vi "Do_ADAM_channel.vi"(4 "Scan Period":dbl format="%.2f", 5 "Previous Scan Value":dbl format="%.2f", 6 "Present scan array":dbl[](array[numeric]) format="%.2f", 7 "Value to Output":dbl format="%.2f", 8 "Ch Description":T1 {"Duty" format="%.0b"; "D" format="%#_5g"; "C" format="%#_5g"; "B" format="%#_5g"; "A" format="%#_5g"}, 9 "Ch names":string[](array[string])) -> (0 "Scan comment":string, 1 "Output":dbl format="%.3f")   [LabVIEW 2014]
uses:
  ADAM Client/Sub VIs/ADAM Controls/Ch_description_ADAM.ctl
  ADAM Client/Sub VIs/ADAM Controls/Module_type_ADAM.ctl
  ADAM Client/Sub VIs/ADAM Controls/Function_ADAM.ctl
  ADAM Client/Sub VIs/ADAM Controls/Channel_State.ctl
  ADAM Client/Sub VIs/ADAM Controls/Calib_type_ADAM.ctl
  ADAM Client/Sub VIs/ADAM Controls/Address.ctl
  ADAM Client/Sub VIs/ADAM Controls/Remember_value_mode.ctl
  ADAM Serial/Instrument drivers/Arduino/ctls_and_globals/Arduino tx msg cluster.ctl
  ADAM Client/Sub VIs/ADAM Controls/Search_mode.ctl
  Anemometry/Anemometry Sub Vis/Controls/In_Range.ctl
  <vilib>/Analysis/baseanly.llb/Mean (DBL).vi
  ADAM_Global.vi
  Anemometry/Anemometry Sub Vis/Globals/Gas_management_global.vi
  Anemometry/Anemometry Sub Vis/Globals/Constants_global.vi
  <vilib>/Analysis/NI_AALBase.lvlib
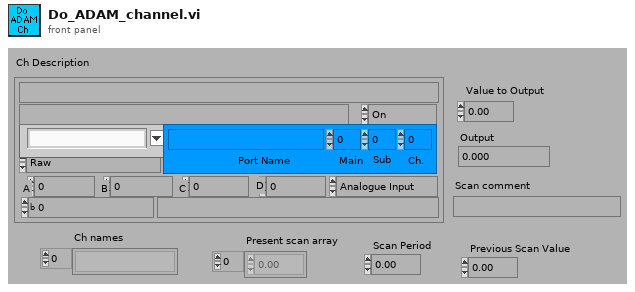
[diagram p1: front panel]
types:
  T1 = typedef "Ch_description_ADAM.ctl" = cluster{"Ch Name":string, "Type":T2, "Function":T3, "Ch State":T4, "Calibration type":T5, "A":dbl, "B":dbl, "C":dbl, "D":dbl, "Comments":string, "Address":T6, "String":string, "Duty":u16}
  T2 = typedef "Module_type_ADAM.ctl" = string
  T3 = typedef "Function_ADAM.ctl" = enum16{"Analogue Input", "Digital Input", "Event counter", "Event rate", "Analogue Output", "Digital Output", "Relay Output"}
  T4 = typedef "Channel_State.ctl" = enum16{"On", "Off", "Always On", "Always Off"}
  T5 = typedef "Calib_type_ADAM.ctl" = enum16{"Raw", "Bx + A", "Cx^2 + Bx + A", "Dx^3 + Cx^2 + Bx + A", "In Band", "Hi-Tec Q", "Hi-Tec M_dot", "Text"}
  T6 = typedef "Address.ctl" = cluster{"Main":i32, "Ch.":i32, "Sub":i32, "Port Name":string}
  T7 = typedef "Remember_value_mode.ctl" = enum16{"Read only", "Read and Write"}
  T8 = typedef "Search_mode.ctl" = enum16{"Between times", "All Times"}
  T9 = typedef "In_Range.ctl" = enum16{"%", "±", "% & ±"}
  T10 = typedef "Arduino tx msg cluster.ctl" = cluster{"dest":u8, "A/D/C/I":string, "R/W":string, "chan":u8, "val (float)":sgl}
  T11 = typedef "Client_State_Cluster.ctl" = cluster{"Client Name":string, "Traverse level State":T12, "People to Email":string[], "Next Contact Time":dbl}
  T12 = typedef "Traverse_Level_State.ctl" = enum16{"Running", "Complete"}
  T13 = cluster{"Centre Times":dbl[], "Output array":dbl[]}
  T14 = cluster{"Centre Times":dbl[], "Output array":dbl[]}[]
  T15 = typedef "Valco_valve_ph.ctl" = u16
  T16 = typedef "LVDateTimeRec.ctl" = cluster{"fractional second":dbl, "second":i32, "minute":i32, "hour":i32, "day of month":i32, "month":i32, "year":i32, "day of week":i32, "day of year":i32, "DST":i32}
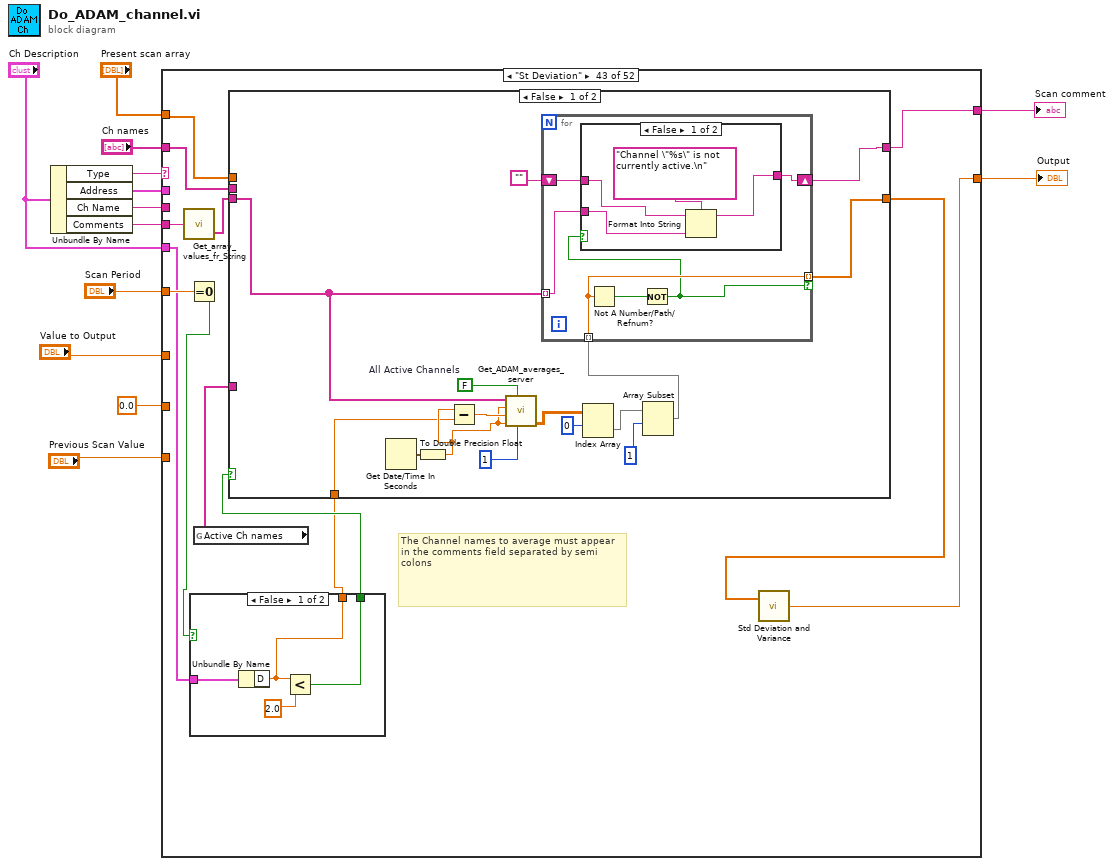
[diagram p0: block diagram]
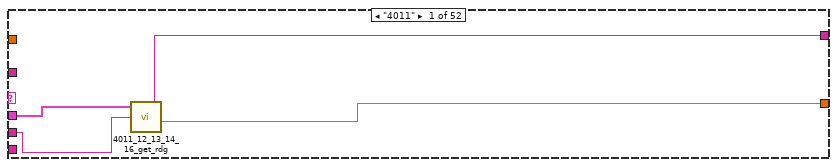
[diagram p2: hidden frame]
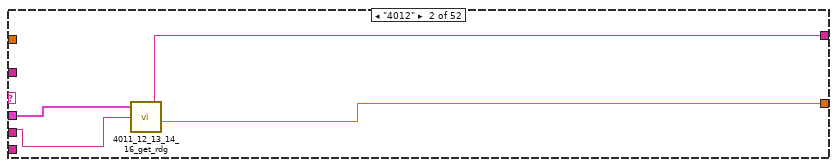
[diagram p3: hidden frame]
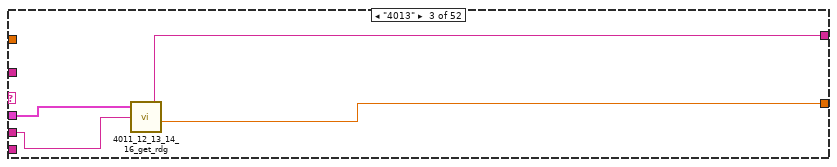
[diagram p4: hidden frame]
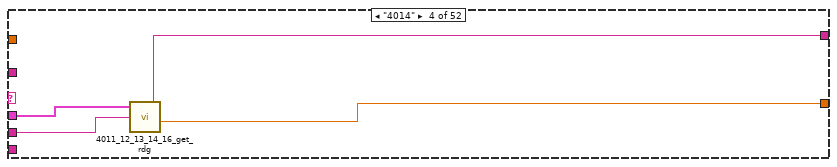
[diagram p5: hidden frame]
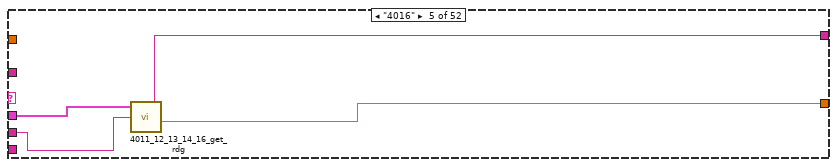
[diagram p6: hidden frame]
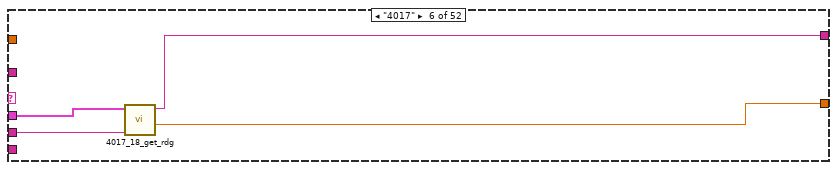
[diagram p7: hidden frame]
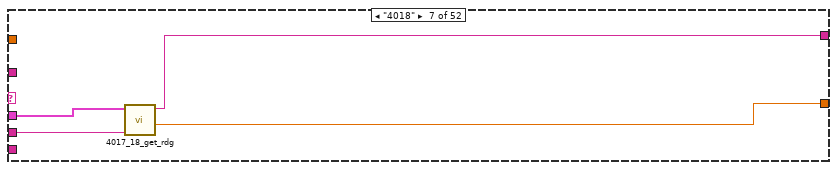
[diagram p8: hidden frame]
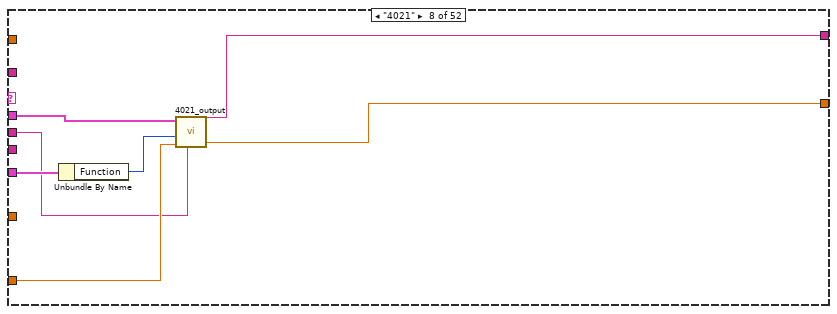
[diagram p9: hidden frame]
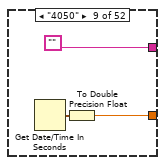
[diagram p10: hidden frame]
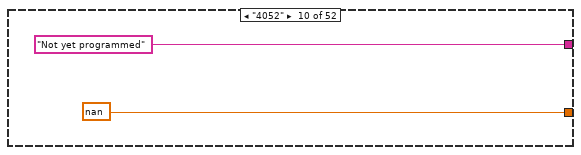
[diagram p11: hidden frame]
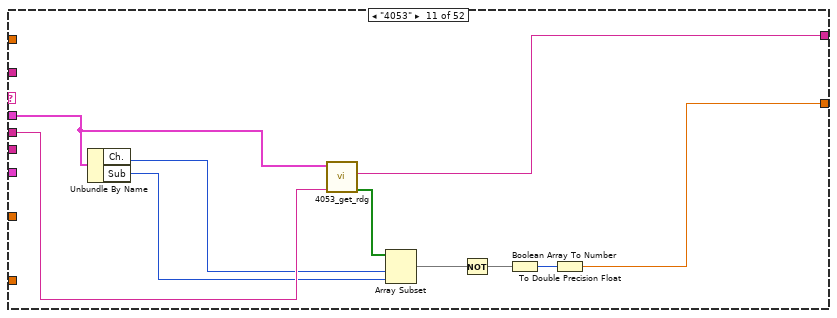
[diagram p12: hidden frame]
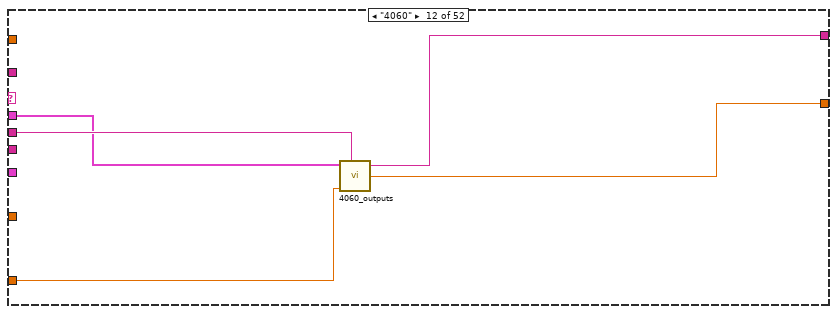
[diagram p13: hidden frame]
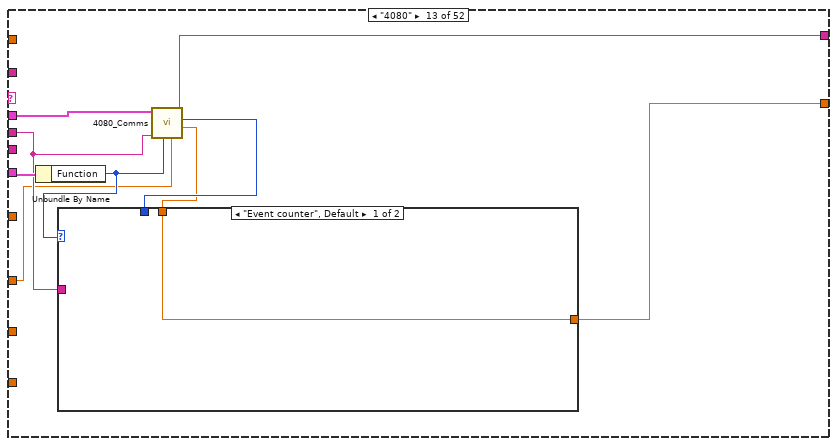
[diagram p14: hidden frame]
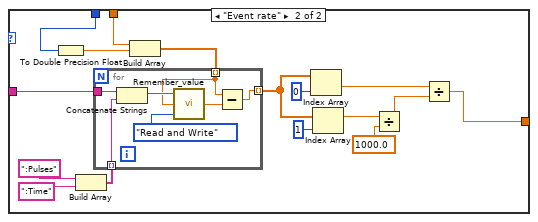
[diagram p15: hidden frame]
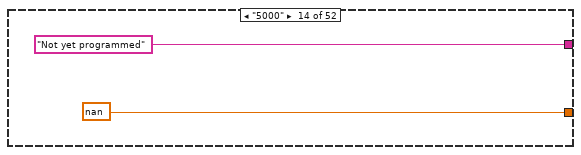
[diagram p16: hidden frame]
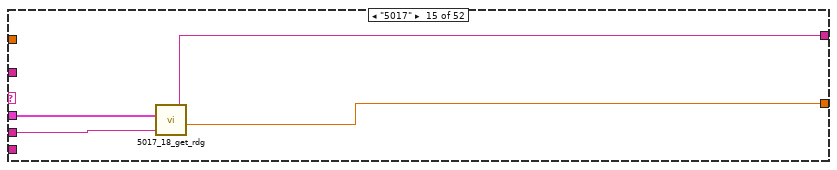
[diagram p17: hidden frame]
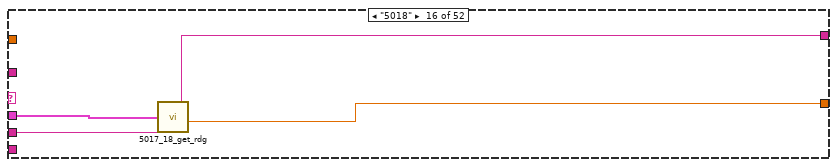
[diagram p18: hidden frame]
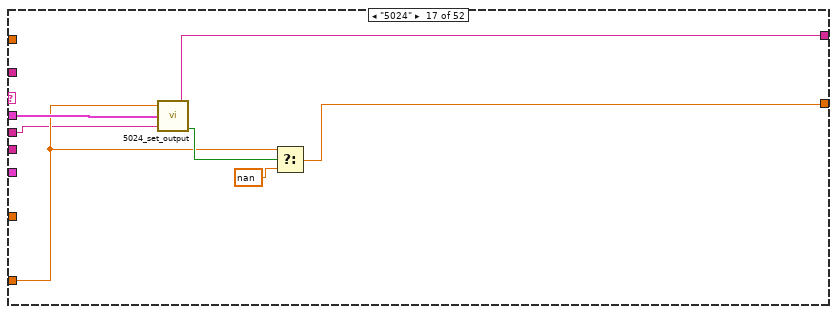
[diagram p19: hidden frame]
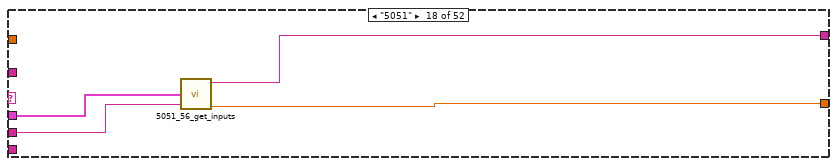
[diagram p20: hidden frame]
diagram:
  n1 = Unbundle By Name("Ch Description") -> ("Type"=w11:T2, "Address"=w10:T6, "Ch Name"=w2:string, "Comments"=w7:string)
  n2 = case shown="\"St Deviation\"" w11 {
    tunnel: [w16 w20 w24 w28 w32 w36 w40 w47 w50 nan w57 w66 w75 nan w105 w109 w114 w120 w128 w149 w171 w190 w205 w221 w250 w270 w358 w371 w373 w375 nan w483 w484 w487 w503 w515 0.0 ("Output") w524 w525 w529 w537 w568 w576 w659 w660 w666 w740 w788 w1279 nan w1310 w1336] -> w8
    tunnel: [w17 w21 w25 w29 w33 w37 w41 w48 "" "Not yet programmed" w62 w67 w77 "Not yet programmed" w106 w110 w117 w121 w127 w150 w172 w189 w208 w223 w245 w267 "" w372 "" w396 "Not yet programmed" w482 "" w488 w502 w516 "Warning; unmatched case in Do_ADAM_channel" ("Status note") w523 "" w530 w536 w567 w570 "Crazy time based random number!" w664 w668 w732 w787 w1280 "Not yet programmed" w1299 ""] -> w5
    tunnel: w10 -> [w14 w18 w22 w26 w30 w34 w38 w42 _ _ w54 w65 w69 _ w107 w111 w118 w122 w126 w151 w173 w204 w220 w236 w261 _ _ w370 _ _ _ w480 _ w486 w505 w518 _ w521 _ _ _ _ _ _ w662 w670 w737 w779 w1285 _ _ w1345]
    tunnel: "Ch Description" -> [_ _ _ _ _ _ _ w46 _ _ _ _ w76 _ _ _ _ _ w125 w148 w170 _ _ _ _ w274 _ _ _ w401 _ _ _ _ _ _ _ _ w526 w531 w542 w569 w574 _ _ w669 _ w781 _ _ _ _]
    tunnel: w2 -> [w15 w19 w23 w27 w31 w35 w39 w43 _ _ w63 w68 w72 _ w104 w108 w112 w119 w123 w145 w167 _ _ _ _ _ w354 _ _ _ _ w481 _ _ w504 w517 _ w522 _ _ _ _ _ _ w663 w667 w733 w784 w1284 _ w1306 _]
    tunnel: "Ch names" -> [_ _ _ _ _ _ _ _ _ _ _ _ _ _ _ _ _ _ _ _ _ _ _ _ _ w279 _ _ _ w400 _ _ _ _ _ _ _ _ _ w532 w543 _ w582 _ _ _ _ w786 _ _ _ _]
    tunnel: "Present scan array" -> [_ _ _ _ _ _ _ _ _ _ _ _ _ _ _ _ _ _ _ _ _ _ _ _ _ w278 _ _ _ w398 _ _ _ _ _ _ _ _ _ w533 w540 _ w581 _ _ _ _ w785 _ _ _ _]
    tunnel: w7 -> [_ _ _ _ _ _ _ _ _ _ _ _ _ _ _ _ _ _ _ _ _ _ _ _ _ w277 _ _ _ w402 _ _ _ _ _ _ _ _ _ _ w535 _ w580 _ _ _ _ _ _ _ _ _]
    tunnel: "Value to Output" -> [_ _ _ _ _ _ _ w44 _ _ _ w64 w70 _ _ _ w113 _ w124 w146 w168 _ w206 w222 _ _ _ _ _ _ _ _ _ _ w501 _ _ _ _ _ w541 _ _ _ _ w665 w741 _ _ _ _ w1340]
    tunnel: "Scan Period" -> [_ _ _ _ _ _ _ _ _ _ _ _ _ _ _ _ _ _ _ _ _ _ _ _ _ w269 _ _ _ _ _ _ _ _ _ _ _ _ _ _ w538 _ w575 _ _ _ _ w783 _ _ _ _]
    tunnel: "Previous Scan Value" -> [_ _ _ _ _ _ _ _ _ _ _ _ _ _ _ _ _ _ _ _ _ w192 _ _ w237 _ _ _ w373 w376 _ _ w484 _ _ _ _ _ _ _ w539 _ _ _ _ _ _ w782 _ _ _ _]
    tunnel: 0.0 -> [_ _ _ _ _ _ _ _ _ _ _ _ _ _ _ _ _ _ _ _ _ _ _ _ _ _ _ _ _ _ _ _ _ _ _ _ _ _ _ _ _ _ _ _ _ _ _ w780 _ _ _ _]
    frame "4011" {
      n3 = call "4011_12_13_14_16_get_rdg.vi"("Address"=w14, "Channel Name"=w15) -> ("Comment"=w17:string, "Reading"=w16:dbl)  [unwired: 1 in, 2 out]
    }
    frame "4012" {
      n4 = call "4011_12_13_14_16_get_rdg.vi"("Address"=w18, "Channel Name"=w19) -> ("Comment"=w21:string, "Reading"=w20:dbl)  [unwired: 1 in, 2 out]
    }
    frame "4013" {
      n5 = call "4011_12_13_14_16_get_rdg.vi"("Address"=w22, "Channel Name"=w23) -> ("Comment"=w25:string, "Reading"=w24:dbl)  [unwired: 1 in, 2 out]
    }
    frame "4014" {
      n6 = call "4011_12_13_14_16_get_rdg.vi"("Address"=w26, "Channel Name"=w27) -> ("Comment"=w29:string, "Reading"=w28:dbl)  [unwired: 1 in, 2 out]
    }
    frame "4016" {
      n7 = call "4011_12_13_14_16_get_rdg.vi"("Address"=w30, "Channel Name"=w31) -> ("Comment"=w33:string, "Reading"=w32:dbl)  [unwired: 1 in, 2 out]
    }
    frame "4017" {
      n8 = call "4017_18_get_rdg.vi"("Channel Name"=w35, "Address"=w34) -> ("Reading"=w36:dbl, "Comment"=w37:string)  [unwired: 2 in, 2 out]
    }
    frame "4018" {
      n9 = call "4017_18_get_rdg.vi"("Channel Name"=w39, "Address"=w38) -> ("Reading"=w40:dbl, "Comment"=w41:string)  [unwired: 2 in, 2 out]
    }
    frame "4021" {
      n10 = Unbundle By Name(w46) -> ("Function"=w45:T3)
      n11 = call "4021_output.vi"("Address"=w42, "Function"=w45, "Set to:"=w44, "Channel Name"=w43) -> ("Comment"=w48:string, "Reading"=w47:dbl)  [unwired: 1 in, 1 out]
    }
    frame "4050" {
      n12 = Get Date/Time In Seconds() -> (seconds since 1Jan1904=w49:timestamp)
      n13 = To Double Precision Float(number=w49) -> (double precision float=w50:dbl)
    }
    frame "4052" {
    }
    frame "4053" {
      n14 = Unbundle By Name(w54) -> ("Ch."=w55:i32, "Sub"=w61:i32)
      n15 = call "4053_get_rdg.vi"("Channel Name"=w63, "Address"=w54) -> ("Boolean array"=w60:bool[], "Comment"=w62:string)  [unwired: 2 in, 2 out]
      n16 = Array Subset(array=w60, index=w55, length=w61) -> (w59:bool[])
      n17 = Not(x=w59) -> (.not. x?=w56:bool[])
      n18 = Boolean Array To Number(Boolean array=w56) -> (number=w58:u32)
      n19 = To Double Precision Float(number=w58) -> (double precision float=w57:dbl)
    }
    frame "4060" {
      n20 = call "4060_outputs.vi"("Address"=w65, "Value to Output"=w64, "Channel Name"=w68) -> ("Comment"=w67:string, "Reading"=w66:dbl)  [unwired: 2 in, 1 out]
    }
    frame "4080" {
      n21 = Unbundle By Name(w76) -> ("Function"=w71:T3)
      n22 = call "4080_Comms.vi"("Value to display"=w70, "Function"=w71, "Channel Name"=w72, "Address"=w69) -> ("Reading"=w73:dbl, "millisecond timer value"=w74:u32, "Comment"=w77:string)  [unwired: 2 in, 1 out]
      n23 = case shown="\"Event counter\", Default" w71 {
        tunnel: w72 -> [_ w94]
        tunnel: w74 -> [_ w87]
        tunnel: [w78 w79] -> w75
        tunnel: w73 -> [w78 w88]
        frame "Event counter", Default {
        }
        frame "Event rate" {
          n24 = To Double Precision Float(number=w87) -> (double precision float=w86:dbl)
          n25 = Build Array(":Pulses", ":Time") -> (w89:string[])
          n26 = Build Array(w88, w86) -> (w85:dbl[])
          n27 = for {
            tunnel: w94 -> [w98]
            tunnel: [w99] -> w82 mode=indexing
            tunnel: w89 -> [w96] mode=indexing
            tunnel: w85 -> [w95] mode=indexing
            n28 = Concatenate Strings(w98, w96) -> (w97:string)
            n29 = call "Remember_value.vi"("Mode"=Remember_value_mode."Read and Write", "Input Value"=w95, "Ch name"=w97) -> ("Output Value"=w100:dbl)
            n30 = Subtract(x=w95, y=w100) -> (x-y=w99:dbl)
          }
          n31 = Index Array(array=w82, index=0) -> (element=w80:dbl)
          n32 = Index Array(array=w82, index=1) -> (element=w81:dbl)
          n33 = Divide(x=w81, y=1000.0) -> (x/y=w92:dbl)
          n34 = Divide(x=w80, y=w92) -> (x/y=w79:dbl)
        }
      }
    }
    frame "5000" {
    }
    frame "5017" {
      n35 = call "5017_18_get_rdg.vi"("Address (all reqd.)"=w107, "Channel Name"=w104) -> ("Comment"=w106:string, "Reading"=w105:dbl)  [unwired: 3 out]
    }
    frame "5018" {
      n36 = call "5017_18_get_rdg.vi"("Address (all reqd.)"=w111, "Channel Name"=w108) -> ("Comment"=w110:string, "Reading"=w109:dbl)  [unwired: 3 out]
    }
    frame "5024" {
      n37 = call "5024_set_output.vi"("Set to:"=w113, "Address (all reqd.)"=w118, "Channel Name"=w112) -> ("Comment"=w117:string, "Good Reply"=w115:bool)  [unwired: 2 out]
      n38 = Select(t=w113, s=w115, f=nan) -> (s? t:f=w114:dbl)
    }
    frame "5051" {
      n39 = call "5051_56_get_inputs.vi"("Address (Main, Sub reqd.)"=w122, "Channel Name"=w119) -> ("Comment"=w121:string, "Single output"=w120:dbl)  [unwired: 3 out]
    }
    frame "5056" {
      n40 = Unbundle By Name(w125) -> ("Function"=w129:T3)
      n41 = case shown="\"Digital Input\"" w129 {
        tunnel: w126 -> [_ w135 w144]
        tunnel: ["This function is not available" w136 w142] -> w127
        tunnel: [nan ("A") w133 w139] -> w128
        tunnel: w124 -> [_ _ w138]
        tunnel: w123 -> [_ w132 w137]
        frame "Analogue Input", Default {
        }
        frame "Digital Input" {
          # "Readback value"
          n42 = call "5060_check_outputs.vi"("Address (Main, Sub reqd.)"=w135, "Channel Name"=w132) -> ("Comment"=w136:string, "Single Channel"=w134:i16)  [unwired: 3 out]
          n43 = To Double Precision Float(number=w134) -> (double precision float=w133:dbl)
        }
        frame "Relay Output" {
          # "Sets single o/p channel"
          n44 = Greater Than 0?(x=w138) -> (x > 0?=w143:bool)
          n45 = call "5056_60_set_single_output.vi"("Channel Name"=w137, "Address (all reqd.)"=w144, "Set state:"=w143) -> ("Comment"=w142:string, "Good Reply"=w141:bool)  [unwired: 2 out]
          n46 = Select(t=w138, s=w141, f=nan) -> (s? t:f=w139:dbl)
        }
      }
    }
    frame "5060" {
      n47 = Unbundle By Name(w148) -> ("Function"=w147:T3)
      n48 = case shown="\"Relay Output\"" w147 {
        tunnel: w151 -> [_ w157 w166]
        tunnel: ["This function is not available" w158 w164] -> w150
        tunnel: [nan ("A") w155 w161] -> w149
        tunnel: w146 -> [_ _ w160]
        tunnel: w145 -> [_ w154 w159]
        frame "Analogue Input", Default {
        }
        frame "Digital Input" {
          # "Readback value"
          n49 = call "5060_check_outputs.vi"("Address (Main, Sub reqd.)"=w157, "Channel Name"=w154) -> ("Comment"=w158:string, "Single Channel"=w156:i16)  [unwired: 3 out]
          n50 = To Double Precision Float(number=w156) -> (double precision float=w155:dbl)
        }
        frame "Relay Output" {
          # "Sets single o/p channel"
          n51 = Greater Than 0?(x=w160) -> (x > 0?=w165:bool)
          n52 = call "5056_60_set_single_output.vi"("Channel Name"=w159, "Address (all reqd.)"=w166, "Set state:"=w165) -> ("Comment"=w164:string, "Good Reply"=w163:bool)  [unwired: 2 out]
          n53 = Select(t=w160, s=w163, f=nan) -> (s? t:f=w161:dbl)
        }
      }
    }
    frame "6060" {
      n54 = Unbundle By Name(w170) -> ("Function"=w169:T3)
      n55 = case shown="\"Digital Input\"" w169 {
        tunnel: w173 -> [_ w179 w188]
        tunnel: ["This function is not available" w180 w186] -> w172
        tunnel: [nan ("A") w177 w183] -> w171
        tunnel: w168 -> [_ _ w182]
        tunnel: w167 -> [_ w176 w181]
        frame "Analogue Input", Default {
        }
        frame "Digital Input" {
          n56 = call "6060_read_all_I-O.vi"("Address (Main, Sub reqd.)"=w179, "Channel Name"=w176) -> ("Comment"=w180:string, "Single Input Channel"=w178:i16)  [unwired: 3 out]
          n57 = To Double Precision Float(number=w178) -> (double precision float=w177:dbl)
        }
        frame "Relay Output" {
          # "Sets single o/p channel"
          n58 = Greater Than 0?(x=w182) -> (x > 0?=w187:bool)
          n59 = call "6060_set_single_output.vi"("Channel Name"=w181, "Address (Main, Ch requd.)"=w188, "Set state:"=w187) -> ("Comment"=w186:string, "Good Reply"=w185:bool)  [unwired: 2 out]
          n60 = Select(t=w182, s=w185, f=nan) -> (s? t:f=w183:dbl)
        }
      }
    }
    frame "Arduino A_in" {
      w198 = T10 {"dest"=1, "A/D/C/I"="A", "R/W"="R", "chan"=1, "val (float)"=0.0}  # Tx msg cluster
      # "Analogue read case"
      n61 = Unbundle By Name(w204) -> ("Port Name"=w195:string, "Main"=w196:i32, "Ch."=w197:i32)
      n62 = To Unsigned Byte Integer(number=w196) -> (unsigned 8bit integer=w203:u8)
      n63 = To Unsigned Byte Integer(number=w197) -> (unsigned 8bit integer=w201:u8)
      n64 = Bundle By Name(cluster=w198, "dest"=w203, "A/D/C/I"="A" ("A/D"), "R/W"="R", "chan"=w201, "val (float)"=sgl 0.0) -> (w194:T10)
      n65 = call "Arduino generic wrapper.vi"("Tx msg cluster"=w194, "Port name"=w195) -> ("Scan comment"=w189:string, "Output"=w191:dbl)
      n66 = Empty String/Path?(string/path=w189) -> (empty?=w193:bool)
      n67 = Select(t=w191, s=w193, f=w192) -> (s? t:f=w190:dbl)
    }
    frame "Arduino A_out" {
      w215 = T10 {"dest"=1, "A/D/C/I"="A", "R/W"="R", "chan"=1, "val (float)"=0.0}  # Tx msg cluster
      # "Analogue write case"
      n68 = Unbundle By Name(w220) -> ("Port Name"=w212:string, "Main"=w213:i32, "Ch."=w214:i32)
      n69 = To Unsigned Byte Integer(number=w213) -> (unsigned 8bit integer=w219:u8)
      n70 = To Unsigned Byte Integer(number=w214) -> (unsigned 8bit integer=w218:u8)
      n71 = To Single Precision Float(number=w206) -> (single precision float=w210:sgl)
      n72 = Bundle By Name(cluster=w215, "dest"=w219, "A/D/C/I"="A" ("A/D"), "R/W"="W", "chan"=w218, "val (float)"=w210) -> (w211:T10)
      n73 = call "Arduino generic wrapper.vi"("Tx msg cluster"=w211, "Port name"=w212) -> ("Scan comment"=w208:string)  [unwired: 1 out]
      n74 = Empty String/Path?(string/path=w208) -> (empty?=w207:bool)
      n75 = Select(t=w206, s=w207, f=nan ("Reading")) -> (s? t:f=w205:dbl)
    }
    frame "Arduino D_out" {
      w231 = T10 {"dest"=1, "A/D/C/I"="A", "R/W"="R", "chan"=1, "val (float)"=0.0}  # Tx msg cluster
      # "Digital write case"
      n76 = Unbundle By Name(w236) -> ("Port Name"=w228:string, "Main"=w229:i32, "Ch."=w230:i32)
      n77 = To Unsigned Byte Integer(number=w229) -> (unsigned 8bit integer=w235:u8)
      n78 = To Unsigned Byte Integer(number=w230) -> (unsigned 8bit integer=w234:u8)
      n79 = To Single Precision Float(number=w222) -> (single precision float=w226:sgl)
      n80 = Bundle By Name(cluster=w231, "dest"=w235, "A/D/C/I"="D" ("A/D"), "R/W"="W", "chan"=w234, "val (float)"=w226) -> (w227:T10)
      n81 = call "Arduino generic wrapper.vi"("Tx msg cluster"=w227, "Port name"=w228) -> ("Scan comment"=w223:string)  [unwired: 1 out]
      n82 = Empty String/Path?(string/path=w223) -> (empty?=w224:bool)
      n83 = Select(t=w222, s=w224, f=nan ("Reading")) -> (s? t:f=w221:dbl)
    }
    frame "Arduino Thermistor" {
      w255 = T10 {"dest"=1, "A/D/C/I"="A", "R/W"="R", "chan"=1, "val (float)"=0.0}  # Tx msg cluster
      # "Thermistor read case"
      # "values not expected in 'normal' operating conditions"
      n84 = Unbundle By Name(w261) -> ("Port Name"=w252:string, "Main"=w253:i32, "Ch."=w254:i32)
      n85 = To Unsigned Byte Integer(number=w253) -> (unsigned 8bit integer=w260:u8)
      n86 = To Unsigned Byte Integer(number=w254) -> (unsigned 8bit integer=w258:u8)
      n87 = Bundle By Name(cluster=w255, "dest"=w260, "A/D/C/I"="A" ("A/D"), "R/W"="R", "chan"=w258, "val (float)"=sgl 0.0) -> (w251:T10)
      n88 = call "Arduino generic wrapper.vi"("Tx msg cluster"=w251, "Port name"=w252) -> ("Scan comment"=w241:string, "Output"=w239:dbl)
      n89 = Empty String/Path?(string/path=w241) -> (empty?=w240:bool)
      n90 = Select(t=w239, s=w240, f=w237) -> (s? t:f=w238:dbl)
      n91 = Less?(x=w239, y=-40.0) -> (x < y?=w242:bool)
      n92 = Greater?(x=w239, y=140.0) -> (0:w243:bool)
      n93 = case shown="False" w242 {
        tunnel: [w263 "Faulty thermistor open-circuit;"] -> w244
        tunnel: w243 -> [w262 _]
        frame False {
          n94 = case shown="True" w262 {
            tunnel: ["" "Faulty thermistor short-circuit;"] -> w263
            frame False {
            }
            frame True {
            }
          }
        }
        frame True {
        }
      }
      n95 = Or(x=w242, y=w243) -> (x .or. y?=w247:bool)
      n96 = Select(t=nan ("f"), s=w247, f=w238) -> (s? t:f=w250:dbl)
      n97 = Concatenate Strings(w241, w244) -> (w245:string)
    }
    frame "Average" {
      # "The Channel names to average must appear in the comments field separated by semi colons"
      n98 = call "Get_array_values_fr_String.vi"("String Value"=w277) -> ("String array"=w276:string[])  [unwired: 1 out]
      n99 = Equal To 0?(x=w269) -> (x = 0?=w268:bool)
      n100 = global read "ADAM_Global.vi" "Active Ch names"() -> (w275:string[])
      n101 = case shown="False" w268 {
        tunnel: w274 -> [w283 _]
        tunnel: [w281 TRUE] -> w273
        tunnel: [w280 2.0 ("A")] -> w272
        frame False {
          n102 = Unbundle By Name(w283) -> ("D"=w280:dbl)
          n103 = Less?(x=w280, y=2.0) -> (x < y?=w281:bool)
        }
        frame True {
        }
      }
      n104 = case shown="True" w273 {
        tunnel: w279 -> [_ w318]
        tunnel: w278 -> [_ w317]
        tunnel: w276 -> [w288 w316]
        tunnel: [w286 w314] -> w267
        tunnel: w275 -> [_ w313]
        tunnel: [w289 w312] -> w271
        tunnel: w272 -> [w290 _]
        frame False {
          w297 = FALSE  # All Active Channels
          n105 = Get Date/Time In Seconds() -> (seconds since 1Jan1904=w300:timestamp)
          n106 = To Double Precision Float(number=w300) -> (double precision float=w298:dbl)
          n107 = Subtract(x=w298, y=w290) -> (x-y=w299:dbl)
          n108 = call "Get_ADAM_averages_server.vi"("No of averages"=1, "All Active Channels"=w297, "End time"=w298, "Start time"=w299, "Clients time"=w298, "ADAM Ch Names"=w288) -> ("DBL values"=w295:dbl[][])  [unwired: 4 out]
          n109 = Index Array(array=w295, index (row)=0) -> (element=w292:dbl[])  [unwired: 1 in]
          n110 = Array Subset(array=w292, index=1) -> (w291:dbl[])  [unwired: 1 in]
          n111 = for {
            tunnel: w291 -> [w306] mode=indexing
            tunnel: [w306] -> w289 mode=indexing if=w304
            tunnel: w288 -> [w303] mode=indexing
            shift-right: [w301] -> w286
            shift-left: "" -> [w302]
            n112 = Not A Number/Path/Refnum?(number/path/refnum=w306) -> (NaN/Path/Refnum?=w305:bool)
            n113 = Not(x=w305) -> (.not. x?=w304:bool)
            n114 = case shown="False" w304 {
              tunnel: w303 -> [w309 _]
              tunnel: w302 -> [w308 w311]
              tunnel: [w307 w311] -> w301
              frame False {
                n115 = Format Into String(format string="Channel \"%s\" is not currently active.\n", initial string=w308, w309) -> (resulting string=w307:string)  [unwired: 1 in, 1 out]
              }
              frame True {
              }
            }
          }
        }
        frame True {
          n116 = for {
            tunnel: w318 -> [w331]
            tunnel: w317 -> [w330]
            tunnel: w316 -> [w327] mode=indexing
            shift-right: [w328] -> w314
            shift-left: "" -> [w329]
            tunnel: [w321] -> w312 mode=indexing if=w319
            tunnel: w313 -> [w322]
            n117 = call "Read_value_of_earlier_Ch.vi"("Desired Ch to Read"=w327, "Ch names"=w331, "Present scan array"=w330) -> ("Value"=w325:dbl, "Scan comment"=w324:string)  [unwired: 1 in]
            n118 = Not A Number/Path/Refnum?(number/path/refnum=w325) -> (NaN/Path/Refnum?=w326:bool)
            n119 = case shown="False" w326 {
              tunnel: w327 -> [w334 _]
              tunnel: [w337 w347] -> w321
              tunnel: w325 -> [w336 w347]
              tunnel: [w339 w346] -> w323
              tunnel: w324 -> [w338 w346]
              tunnel: w322 -> [w335 _]
              frame False {
                n120 = Search 1D Array(1D array=w335, element=w334) -> (index of element=w332:i32)  [unwired: 1 in]
                n121 = Greater Or Equal To 0?(x=w332) -> (x >= 0?=w333:bool)
                n122 = case shown="False" w333 {
                  tunnel: w334 -> [w343 _]
                  tunnel: [w342 w345] -> w339
                  tunnel: w338 -> [_ w345]
                  tunnel: [nan w344] -> w337
                  tunnel: w336 -> [_ w344]
                  frame False {
                    n123 = Format Into String(format string="Channel \"%s\" is not currently active.\n", w343) -> (resulting string=w342:string)  [unwired: 2 in, 1 out]
                  }
                  frame True {
                  }
                }
              }
              frame True {
              }
            }
            n124 = Concatenate Strings(w329, w323) -> (w328:string)
            n125 = Not A Number/Path/Refnum?(number/path/refnum=w321) -> (NaN/Path/Refnum?=w320:bool)
            n126 = Not(x=w320) -> (.not. x?=w319:bool)
          }
        }
      }
      n127 = call-poly <vilib>:"Mean.vi"("X"=w271) -> ("mean"=w270:dbl)  [unwired: 1 out]
    }
    frame "Client Info" {
      n128 = global read "ADAM_Global.vi" "Client State Array"() -> (w360:T11[])
      n129 = call "Split_Ch_name.vi"("Ch name"=w354) -> ("Top level"=w352:string, "Low level"=w350:string)  [unwired: 1 out]
      n130 = Equal?(x="Status" ("Substring"), y=w352) -> (x = y?=w351:bool)
      n131 = Select(t=w350, s=w351, f="") -> (s? t:f=w348:string)
      n132 = for {
        tunnel: w360 -> [w369] mode=indexing
        tunnel: [w368] -> w361 mode=indexing
        n133 = Unbundle By Name(w369) -> ("Client Name"=w368:string)
      }
      n134 = Search 1D Array(1D array=w361, element=w348) -> (index of element=w356:i32)  [unwired: 1 out]
      n135 = Less Than 0?(x=w356) -> (x < 0?=w355:bool)
      n136 = Index Array(array=w360, index=w356) -> (element=w359:T11)
      n137 = case shown="False" w355 {
        tunnel: w359 -> [w364 _]
        tunnel: w348 -> [w363 w366]
        tunnel: [w362 w365] -> w358
        frame False {
          n138 = call "Get_Client_Status_string.vi"("Client State Cluster"=w364, "Client Name"=w363) -> ("Code Value"=w362:dbl)  [unwired: 1 in]
        }
        frame True {
          w365 = 7.0 ("Code Value")
          n139 = call "Remember_value.vi"("Mode"=Remember_value_mode."Read and Write", "Input Value"=w365, "Ch name"=w366) -> ()  [unwired: 1 out]
        }
      }
    }
    frame "ClimatronicsUDP" {
      n140 = call "ClimatronicsUDP_get_rdg.vi"("Address"=w370) -> ("Output"=w371:dbl, "Status note"=w372:string)  [unwired: 5 in]
    }
    frame "Coded" {
    }
    frame "Comparator" {
      # "A Warn if above this value\nB Warn if below this value\nC  Hysteresis margin\nD is the averaging time in minutes\nComments   is Channel name to check"
      n141 = Unbundle By Name(w401) -> ("D"=w384:dbl)
      n142 = Match Pattern(string=w402, regular expression=":::" ("String to match")) -> (before substring=w399:string)  [unwired: 4 out]
      n143 = call "Read_value_of_earlier_Ch.vi"("Desired Ch to Read"=w399, "Ch names"=w400, "Present scan array"=w398) -> ("Value"=w383:dbl, "Scan comment"=w397:string)  [unwired: 1 in]
      n144 = Equal?(x=w376, y=1.0) -> (x = y?=w392:bool)
      n145 = Unbundle By Name(w401) -> ("A"=w395:dbl, "B"=w394:dbl, "C"=w393:dbl)
      n146 = Equal To 0?(x=w384) -> (x = 0?=w382:bool)
      n147 = case shown="True" w392 {
        tunnel: [w408 w413] -> w390
        tunnel: w395 -> [w408 w412]
        tunnel: w394 -> [w407 w411]
        tunnel: [w407 w409] -> w391
        tunnel: w393 -> [_ w410]
        frame False {
        }
        frame True {
          n148 = Subtract(x=w412, y=w410) -> (x-y=w413:dbl)
          n149 = Add(x=w411, y=w410) -> (x+y=w409:dbl)
        }
      }
      n150 = case shown="False" w382 {
        tunnel: [w418 w421] -> w405
        tunnel: w399 -> [w420 _]
        tunnel: [w416 w422] -> w381
        tunnel: w384 -> [w414 _]
        tunnel: w383 -> [_ w422]
        tunnel: w397 -> [w418 w421]
        frame False {
          n151 = Build Array(w420) -> (w415:string[])
          n152 = call "Get_Channel_averages.vi"("Desired Ch Names"=w415, "Averaging time (mins)"=w414) -> ("number"=w417:dbl[])  [unwired: 1 in, 2 out]
          n153 = Index Array(array=w417, index=0) -> (element=w416:dbl)
        }
        frame True {
        }
      }
      n154 = Not(x=w392) -> (.not. x?=w385:bool)
      n155 = In Range and Coerce(upper limit=w390, x=w381, lower limit=w391) -> (In Range?=w386:bool)  [unwired: 1 out]
      n156 = Greater?(x=w381, y=w390) -> (0:w389:bool)
      n157 = Not A Number/Path/Refnum?(number/path/refnum=w381) -> (NaN/Path/Refnum?=w378:bool)
      n158 = Equal?(x=w386, y=w385) -> (x = y?=w380:bool)
      n159 = Or(x=w380, y=w378) -> (x .or. y?=w379:bool)
      n160 = case shown="False" w379 {
        tunnel: w399 -> [w429 _]
        tunnel: w390 -> [w428 _]
        tunnel: w401 -> [w427 _]
        tunnel: w391 -> [w426 _]
        tunnel: w386 -> [w425 _]
        tunnel: w381 -> [w424 _]
        tunnel: w389 -> [w423 _]
        frame False {
          n161 = stacked-sequence {
            seq-local: [w435 _ _ _ _] -> [_ _ _ w476 _]
            seq-local: [_ w455 _ _ _] -> [_ _ _ w473 _]
            seq-local: [w433 _ _ _ _] -> [_ _ _ w469 _]
            tunnel: w429 -> [w437 w463 _ w475 _]
            tunnel: w428 -> [w436 _ _ _ _]
            tunnel: w427 -> [_ _ w468 w477 _]
            tunnel: w426 -> [w434 _ _ _ _]
            tunnel: w425 -> [w432 _ _ _ _]
            tunnel: w424 -> [w431 _ _ _ _]
            tunnel: w423 -> [w430 _ _ _ _]
            frame #0 {
              n162 = case shown="True" w432 {
                tunnel: w437 -> [w442 w453]
                tunnel: w436 -> [_ w446]
                tunnel: [w440 w452] -> w435
                tunnel: w434 -> [_ w445]
                tunnel: ["OK " ""] -> w433
                tunnel: w431 -> [w438 _]
                tunnel: w430 -> [_ w443]
                frame True {
                  n163 = Format Into String(format string="The channel named %s is now  %.3f" ("Format String"), w442, w438) -> (resulting string=w440:string)  [unwired: 2 in, 1 out]
                }
                frame False {
                  n164 = Select(t=w446, s=w443, f=w445) -> (s? t:f=w444:dbl)
                  n165 = Select(t="greater", s=w443, f="less") -> (s? t:f=w448:string)
                  n166 = Format Into String(format string="%s is %s than %.3f" ("Format String"), w453, w448, w444) -> (resulting string=w452:string)  [unwired: 2 in, 1 out]
                }
              }
            }
            frame #1 {
              n167 = Build Array(w463) -> (w462:string[])
              n168 = call "Channel_Names_and_indicies.vi"("All Active Channels"=FALSE, "Desired Ch Names"=w462) -> ("Indicies"=w460:i32[])  [unwired: 1 out]
              n169 = call "Specified_Channels_server.vi"("Mode"=Search_mode."All Times", "Requested channels"=w460) -> ("Output array"=w458:dbl[][], "Centre Times"=w454:dbl[])  [unwired: 3 in, 3 out]
              n170 = Index Array(array=w458, index (row)=0) -> (element=w456:dbl[])  [unwired: 1 in]
              n171 = Bundle("Centre Times"=w454, "Output array"=w456) -> (w459:T13)  [unwired: 1 out]
              n172 = Build Array(w459) -> (w455:T14)
            }
            frame #2 {
              w466 = TRUE  # Contact All clients?
              n173 = Unbundle By Name(w468) -> ("String"=w467:string)
              n174 = call "Get_array_values_fr_String.vi"("String Value"=w467) -> ("String array"=w465:string[])  [unwired: 1 out]
              n175 = call "Client_email_addresses.vi"("Extra People to Email"=w465, "Contact All clients?"=w466) -> ()  [unwired: 1 in]
            }
            frame #3 {
              n176 = Unbundle By Name(w477) -> ("Ch Name"=w470:string)
              n177 = Build Array(w475) -> (w474:string[])
              n178 = Concatenate Strings(w469, w470) -> (w471:string)
              n179 = call "Email_Attachment_Plot.vi"("X axis name"="Time", "XY Graph"=w473, "Series Names"=w474, "message"=w476, "subject ([No Subject])"=w471) -> ()  [unwired: 1 in, 1 out]
            }
            frame #4 {
            }
          }
        }
        frame True {
        }
      }
      n180 = Concatenate Strings(w405, "") -> (w396:string)
      n181 = Select(t=0.0, s=w386, f=1.0) -> (s? t:f=w377:dbl)
      n182 = Select(t=w376, s=w378, f=w377) -> (s? t:f=w375:dbl)
    }
    frame "DRUCK" {
    }
    frame "GILL" {
      n183 = call "Gill_get_rdg.vi"("Channel Name"=w481, "Address"=w480) -> ("Output"=w483:dbl, "Status note"=w482:string)  [unwired: 2 in, 2 out]
    }
    frame "Hold Value" {
    }
    frame "IR2100" {
      n184 = call "IR2100_get_rdg.vi"("Address"=w486) -> ("Comment"=w488:string, "Reading"=w487:dbl)  [unwired: 2 in, 2 out]
    }
    frame "JEM" {
      n185 = Unbundle By Name(w505) -> ("Main"=w491:i32, "Ch."=w490:i32, "Port Name"=w500:string)
      n186 = case shown="0, Default" w490 {
        tunnel: [i16[] [-3, -2, -1, 0, 14, 29, 43, 57, 71, 86, 100] i16[] [0, 20, 40, 60, 80, 100, 120]] -> w494
        tunnel: [u8[] [10, 50, 80, 100, 120, 140, 160, 180, 200, 220, 240] u8[] [20, 50, 90, 130, 160, 200, 230]] -> w495
        frame 0, Default {
        }
        frame 1 {
        }
      }
      n187 = Add(x=w491, y=w490) -> (x+y=w489:i32)
      n188 = Threshold 1D Array(2:w501, 3:w494) -> (0:w497:dbl)  [unwired: 1 out]
      n189 = Round To Nearest(number=w497) -> (nearest integer value=w498:dbl)
      n190 = To Long Integer(number=w498) -> (32bit integer=w496:i32)
      n191 = Index Array(array=w495, index=w496) -> (element=w493:u8)
      n192 = call "DMX.vi"("Port Name"=w500, "DMX channel no."=w489, "Set value:"=w493, "Channel Name"=w504) -> ("error"=w499:bool)  [unwired: 2 out]
      n193 = Index Array(array=w494, index=w496) -> (element=w492:i16)
      n194 = case shown="False" w499 {
        tunnel: [w506 nan] -> w503
        tunnel: ["" "Comms Error"] -> w502
        tunnel: w492 -> [w508 _]
        frame False {
          n195 = To Double Precision Float(number=w508) -> (double precision float=w506:dbl)
        }
        frame True {
        }
      }
    }
    frame "LPA" {
      # "LPA was, IIRC, a serially-polled weighing platform we rented at Surrey for Athena Scaperdas' project at Atkins to weigh a helicopter with rotor running. \nTo add to the fun, it was RS232, so to make it addressable it was polled through an addressable ADAM 485-232 module"
      n196 = call "LPA400_get_rdg.vi"("Channel Name"=w517, "Address"=w518) -> ("Output"=w515:dbl, "Status note"=w516:string)  [unwired: 4 out]
    }
    frame "Oops", Default {
    }
    frame "PPT" {
      n197 = call "PPT_get_rdg.vi"("Channel Name"=w522, "Address"=w521) -> ("Reading"=w524:dbl, "Comment"=w523:string)  [unwired: 2 in, 2 out]
    }
    frame "Read A" {
      n198 = Unbundle By Name(w526) -> ("A"=w525:dbl)
    }
    frame "Read Ch" {
      n199 = Unbundle By Name(w531) -> ("String"=w528:string)
      n200 = call "Read_value_of_earlier_Ch.vi"("Desired Ch to Read"=w528, "Ch names"=w532, "Present scan array"=w533) -> ("Value"=w529:dbl, "Scan comment"=w530:string)  [unwired: 1 in]
    }
    frame "Run VI Named:" {
      n201 = Current VI's Path() -> (path=w552:path)
      n202 = Strip Path(path=w552) -> (stripped path=w553:path)  [unwired: 1 out]
      n203 = call <vilib>:"Trim Whitespace.vi"("string"=w535) -> ("trimmed string"=w534:string)  [unwired: 1 in]
      n204 = Strip Path(path=w553) -> (stripped path=w554:path)  [unwired: 1 out]
      n205 = Build Path(base path=w554, name or relative path="Run_vi_named") -> (appended path=w556:path)
      n206 = Build Path(base path=w556, name or relative path=w534) -> (appended path=w551:path)
      n207 = Open VI Reference(type specifier VI Refnum (for type only)=refnum<vi> refnum, vi path=w551) -> (vi reference=w547:refnum<vi>, error out=w546:errorcluster)  [unwired: 1 in, 3 out]
      n208 = property class="VI Interface Type 0"(reference=w547, error in=w546) -> (reference out=w549:refnum<vi>, error out=w548:errorcluster, "Front Panel Window:Open"=w550:bool)
      n209 = case shown="False" w550 {
        tunnel: w549 -> [w564 w566]
        tunnel: w548 -> [w563 w565]
        tunnel: [w562 w566] -> w545
        tunnel: [w560 w565] -> w544
        frame False {
          n210 = property class="VI Interface Type 0"(reference=w564, error in=w563, "Front Panel Window:Open"=TRUE) -> (reference out=w562:refnum<vi>, error out=w560:errorcluster)
        }
        frame True {
        }
      }
      n211 = call-by-ref "?"(reference=w545, error in=w544, "Scan Period"=w538, "Previous Scan Value"=w539, "Present scan array"=w540, "Value to Output"=w541, "Ch Description"=w542, "Ch names"=w543) -> (reference out=w558:refnum<vi>, error out=w559:errorcluster, "Scan comment"=w536:string, "Output"=w537:dbl)  [unwired: 2 in]
      n212 = Close Reference(reference=w558, error in (no error)=w559) -> ()  [unwired: 1 out]
    }
    frame "ScanPacer" {
      # "Uses a metronome to slow an otherwise over-fast scan table"
      n213 = call "ADAMPacer.vi"("Ch Description"=w569) -> ("Scan comment"=w567:string, "Output"=w568:dbl)  [unwired: 7 in]
    }
    frame "St Deviation" {
      # "The Channel names to average must appear in the comments field separated by semi colons"
      n214 = call "Get_array_values_fr_String.vi"("String Value"=w580) -> ("String array"=w579:string[])  [unwired: 1 out]
      n215 = Equal To 0?(x=w575) -> (x = 0?=w573:bool)
      n216 = case shown="False" w573 {
        tunnel: w574 -> [w586 _]
        tunnel: [w584 TRUE] -> w572
        tunnel: [w583 2.0 ("A")] -> w571
        frame False {
          n217 = Unbundle By Name(w586) -> ("D"=w583:dbl)
          n218 = Less?(x=w583, y=2.0) -> (x < y?=w584:bool)
        }
        frame True {
        }
      }
      n219 = global read "ADAM_Global.vi" "Active Ch names"() -> (w578:string[])
      n220 = case shown="False" w572 {
        tunnel: w582 -> [_ w621]
        tunnel: w581 -> [_ w620]
        tunnel: w579 -> [w591 w619]
        tunnel: [w589 w617] -> w570
        tunnel: w578 -> [_ w616]
        tunnel: [w592 w615] -> w577
        tunnel: w571 -> [w593 _]
        frame False {
          w600 = FALSE  # All Active Channels
          n221 = Get Date/Time In Seconds() -> (seconds since 1Jan1904=w603:timestamp)
          n222 = To Double Precision Float(number=w603) -> (double precision float=w601:dbl)
          n223 = Subtract(x=w601, y=w593) -> (x-y=w602:dbl)
          n224 = call "Get_ADAM_averages_server.vi"("No of averages"=1, "All Active Channels"=w600, "End time"=w601, "Start time"=w602, "Clients time"=w601, "ADAM Ch Names"=w591) -> ("DBL values"=w598:dbl[][])  [unwired: 4 out]
          n225 = Index Array(array=w598, index (row)=0) -> (element=w595:dbl[])  [unwired: 1 in]
          n226 = Array Subset(array=w595, index=1) -> (w594:dbl[])  [unwired: 1 in]
          n227 = for {
            tunnel: w594 -> [w609] mode=indexing
            tunnel: [w609] -> w592 mode=indexing if=w607
            tunnel: w591 -> [w606] mode=indexing
            shift-right: [w604] -> w589
            shift-left: "" -> [w605]
            n228 = Not A Number/Path/Refnum?(number/path/refnum=w609) -> (NaN/Path/Refnum?=w608:bool)
            n229 = Not(x=w608) -> (.not. x?=w607:bool)
            n230 = case shown="False" w607 {
              tunnel: w606 -> [w612 _]
              tunnel: w605 -> [w611 w614]
              tunnel: [w610 w614] -> w604
              frame False {
                n231 = Format Into String(format string="Channel \"%s\" is not currently active.\n", initial string=w611, w612) -> (resulting string=w610:string)  [unwired: 1 in, 1 out]
              }
              frame True {
              }
            }
          }
        }
        frame True {
          n232 = for {
            tunnel: w621 -> [w634]
            tunnel: w620 -> [w633]
            tunnel: w619 -> [w630] mode=indexing
            shift-right: [w631] -> w617
            shift-left: "" -> [w632]
            tunnel: [w624] -> w615 mode=indexing if=w622
            tunnel: w616 -> [w625]
            n233 = call "Read_value_of_earlier_Ch.vi"("Desired Ch to Read"=w630, "Ch names"=w634, "Present scan array"=w633) -> ("Value"=w628:dbl, "Scan comment"=w627:string)  [unwired: 1 in]
            n234 = Not A Number/Path/Refnum?(number/path/refnum=w628) -> (NaN/Path/Refnum?=w629:bool)
            n235 = case shown="False" w629 {
              tunnel: w630 -> [w637 _]
              tunnel: [w640 w650] -> w624
              tunnel: w628 -> [w639 w650]
              tunnel: [w642 w649] -> w626
              tunnel: w627 -> [w641 w649]
              tunnel: w625 -> [w638 _]
              frame False {
                n236 = Search 1D Array(1D array=w638, element=w637) -> (index of element=w635:i32)  [unwired: 1 in]
                n237 = Greater Or Equal To 0?(x=w635) -> (x >= 0?=w636:bool)
                n238 = case shown="False" w636 {
                  tunnel: w637 -> [w646 _]
                  tunnel: [w645 w648] -> w642
                  tunnel: w641 -> [_ w648]
                  tunnel: [nan w647] -> w640
                  tunnel: w639 -> [_ w647]
                  frame False {
                    n239 = Format Into String(format string="Channel \"%s\" is not currently active.\n", w646) -> (resulting string=w645:string)  [unwired: 2 in, 1 out]
                  }
                  frame True {
                  }
                }
              }
              frame True {
              }
            }
            n240 = Concatenate Strings(w632, w626) -> (w631:string)
            n241 = Not A Number/Path/Refnum?(number/path/refnum=w624) -> (NaN/Path/Refnum?=w623:bool)
            n242 = Not(x=w623) -> (.not. x?=w622:bool)
          }
        }
      }
      n243 = call <vilib>:"Std Deviation and Variance.vi"("X"=w577) -> ("standard deviation"=w576:dbl)  [unwired: 1 in, 2 out]
    }
    frame "Test" {
      w654 = 0.0005  # y
      n244 = Get Date/Time In Seconds() -> (seconds since 1Jan1904=w651:timestamp)
      n245 = To Double Precision Float(number=w651) -> (double precision float=w656:dbl)
      n246 = Subtract(x=w656, y=2969882881.0) -> (x-y=w655:dbl)
      n247 = Multiply(x=w655, y=w654) -> (x*y=w652:dbl)
      n248 = Random Number (0-1)() -> (number: 0 to 1=w653:dbl)
      n249 = Add(x=w653, y=w652) -> (x+y=w659:dbl)
    }
    frame "Thermistor" {
      n250 = call "4017_18_get_rdg.vi"("Channel Name"=w663, "Address"=w662) -> ("Reading"=w661:dbl, "Comment"=w664:string)  [unwired: 2 in, 2 out]
      n251 = call "Thermistor volts to temperature.vi"("V2 (V)"=w661) -> ("Temperature (degC)"=w660:dbl)
    }
    frame "Tracker" {
      n252 = while {
        tunnel: w670 -> [w694]
        tunnel: w669 -> [w693]
        tunnel: [w687] -> w668
        tunnel: w667 -> [w686]
        tunnel: [w680] -> w666
        tunnel: w665 -> [w679]
        i -> [w676]
        stop <- w673 continue-if-true
        n253 = Unbundle By Name(w693) -> ("Function"=w692:T3)
        n254 = Unbundle By Name(w694) -> ("Port Name"=w691:string, "Ch."=w682:i32, "Main"=w690:i32, "Sub"=w689:i32)
        n255 = case shown="\"Analogue Output\"" w692 {
          tunnel: [enum16{"Set", "Read"}."Set" ("Set") enum16{"Set", "Read"}."Set" ("Set") enum16{"Set", "Read"}."Set" ("Set") enum16{"Set", "Read"}."Set" ("Set") enum16{"Set", "Read"}."Set" ("Set") enum16{"Set", "Read"}."Read" ("Set") enum16{"Set", "Read"}."Read" ("Set")] -> w677
          tunnel: [enum16{"Logic", "Analogue"}."Analogue" ("Analogue") enum16{"Logic", "Analogue"}."Logic" ("Analogue") enum16{"Logic", "Analogue"}."Logic" ("Analogue") enum16{"Logic", "Analogue"}."Logic" ("Analogue") enum16{"Logic", "Analogue"}."Logic" ("Analogue") enum16{"Logic", "Analogue"}."Logic" ("Analogue") enum16{"Logic", "Analogue"}."Analogue" ("Analogue")] -> w688
          frame "Analogue Output" {
          }
          frame "Digital Output" {
          }
          frame "Relay Output" {
          }
          frame "Event rate" {
          }
          frame "Event counter" {
          }
          frame "Digital Input" {
          }
          frame "Analogue Input" {
          }
        }
        n256 = call "TalkTracker.vi"("PORT NAME"=w691, "Set"=w677, "Channel Name"=w686, "Value to set"=w679, "MODULE ADDRESS"=w690, "LOCATION"=w682, "NO. LOCATIONS"=w689, "Analogue"=w688) -> ("Response"=w684:string, "Good Set?"=w671:bool, "Comment out"=w687:string)  [unwired: 1 in, 4 out]
        n257 = Match Pattern(string=w684, regular expression="\r\n") -> (before substring=w683:string)  [unwired: 4 out]
        n258 = case shown="\"Set\"" w677 {
          tunnel: w683 -> [_ w706]
          tunnel: [w698 w705] -> w681
          tunnel: w679 -> [w700 _]
          tunnel: nan ("Reading") -> [w699 w704]
          tunnel: [w697 w702] -> w674
          tunnel: [0 ("y") 1 ("y")] -> w672
          tunnel: w671 -> [w695 _]
          frame "Set" {
            n259 = Not(x=w695) -> (.not. x?=w697:bool)
            n260 = Select(t=w700, s=w695, f=w699) -> (s? t:f=w698:dbl)
          }
          frame "Read" {
            n261 = String Length(string=w706) -> (length=w708:i32)
            n262 = Fract/Exp String To Number(string=w706, default (0 dbl)=w704) -> (offset past number=w709:i32, number=w707:dbl)  [unwired: 2 out]
            n263 = Equal?(x=w708, y=w709) -> (x = y?=w703:bool)
            n264 = Not(x=w703) -> (.not. x?=w702:bool)
            n265 = Select(t=w707, s=w703, f=w704) -> (s? t:f=w705:dbl)
          }
        }
        n266 = case shown="0, Default" w682 {
          tunnel: w681 -> [w710 w713]
          tunnel: [w710 w711] -> w680
          frame 0, Default {
          }
          frame 283 {
            n267 = Equal To 0?(x=w713) -> (x = 0?=w714:bool)
            n268 = Select(t=nan ("Reading"), s=w714, f=w713) -> (s? t:f=w711:dbl)
          }
        }
        n269 = Less?(x=w676, y=w672) -> (x < y?=w675:bool)
        n270 = And(x=w674, y=w675) -> (x .and. y?=w673:bool)
      }
    }
    frame "VICI" {
      n271 = To Long Integer(number=w741) -> (32bit integer=w736:i32)
      n272 = Unbundle By Name(w737) -> ("Port Name"=w739:string, "Ch."=w738:i32)
      n273 = call "Valco_Valve_Position.vi"("Channel Name"=w733, "Valve Number"=w738, "Port Name"=w739, "Requested Posn."=w736) -> ("Error Message"=w731:string, "Achieved Posn."=w734:T15)  [unwired: 2 out]
      n274 = Empty String/Path?(string/path=w731) -> ()  [unwired: 1 out]
      n275 = case shown="True" TRUE {
        tunnel: w737 -> [w748 _]
        tunnel: w736 -> [w747 _]
        tunnel: [w746 w778] -> w735
        tunnel: w734 -> [_ w778]
        tunnel: w733 -> [w745 _]
        tunnel: [w744 w777] -> w732
        tunnel: w731 -> [_ w777]
        tunnel: w731 -> [w743 _]
        tunnel: "X10" ("Port Name") -> [w742 _]
        frame False {
          n276 = stacked-sequence {
            tunnel: w748 -> [_ _ _ _ _ w769]
            tunnel: w747 -> [_ _ _ _ _ w765]
            tunnel: [_ _ _ _ _ w768] -> w746
            tunnel: w745 -> [_ _ _ _ _ w767]
            tunnel: [_ _ _ _ _ w766] -> w744
            tunnel: w743 -> [_ w754 _ _ _ _]
            tunnel: w742 -> [w749 _ _ w757 _ _]
            frame #0 {
              w751 = 3 items=["-----", "A", "B", "C", "D", "E", "F", "G", "H", "I", "J", "K", "L", "M", "N", "O", "P"] ("House Code")
              n277 = call "X10control.vi"("Port Name"=w749, "Power Request (ON)"=FALSE, "House Code"=w751, "Unit No."=5) -> ()  [unwired: 6 out]
            }
            frame #1 {
              n278 = call "Server_Emails.vi"("Message"=w754, "Contact All clients?"=TRUE, "Subject"="Powering Down FID Valve" ("Error Type")) -> ()  [unwired: 2 in, 3 out]
            }
            frame #2 {
              n279 = Wait (ms)(milliseconds to wait=u32 20000) -> ()  [unwired: 1 out]
            }
            frame #3 {
              w759 = 3 items=["-----", "A", "B", "C", "D", "E", "F", "G", "H", "I", "J", "K", "L", "M", "N", "O", "P"] ("House Code")
              n280 = call "X10control.vi"("Port Name"=w757, "Power Request (ON)"=TRUE, "House Code"=w759, "Unit No."=5) -> ()  [unwired: 6 out]
            }
            frame #4 {
              n281 = Wait (ms)(milliseconds to wait=u32 5000) -> ()  [unwired: 1 out]
            }
            frame #5 {
              n282 = Build Array(1 ("element"), 2 ("element"), w765) -> (w762:i32[])
              n283 = for {
                tunnel: w769 -> [w774]
                tunnel: [w773] -> w768
                tunnel: w767 -> [w772]
                tunnel: [w771] -> w766
                tunnel: w762 -> [w770] mode=indexing
                n284 = Unbundle By Name(w774) -> ("Port Name"=w775:string, "Ch."=w776:i32)
                n285 = call "Valco_Valve_Position.vi"("Channel Name"=w772, "Valve Number"=w776, "Port Name"=w775, "Requested Posn."=w770) -> ("Error Message"=w771:string, "Achieved Posn."=w773:T15)  [unwired: 2 out]
              }
            }
          }
        }
        frame True {
        }
      }
      n286 = To Double Precision Float(number=w735) -> (double precision float=w740:dbl)
    }
    frame "VIRTUAL" {
      n287 = case shown="\"EnFlo_Tunnel:Days Run at:2.5m/s\"" w784 {
        tunnel: [w798 w812 w826 w848 w863 w874 w890 w918 w946 w1030 w1040 w1076 w1129 w1155 w1182 w1202] -> w788
        tunnel: [w789 w818 w824 w852 w857 w872 w899 w922 w947 w1024 w1046 w1073 w1128 w1154 "" w1203] -> w787
        tunnel: w786 -> [w795 w820 w830 w854 w859 w877 w901 w924 w949 w1026 w1036 w1074 w1134 w1159 _ w1205]
        tunnel: w785 -> [w796 w819 w831 w853 w858 w878 w900 w925 w950 w1025 w1037 w1075 w1136 w1161 _ w1204]
        tunnel: w784 -> [w793 _ _ _ _ _ _ _ _ _ _ w1062 _ _ w1177 _]
        tunnel: w783 -> [w794 _ _ _ _ _ _ _ _ _ _ _ w1126 w1153 w1182 w1201]
        tunnel: w782 -> [w797 _ _ _ _ _ _ _ _ _ _ w1077 w1130 w1156 _ w1200]
        tunnel: w781 -> [_ _ w822 _ _ _ _ _ w951 _ _ w1068 _ _ _ _]
        tunnel: w780 -> [_ w811 _ _ _ w871 _ _ _ _ _ _ _ _ _ _]
        tunnel: w779 -> [_ _ _ _ _ _ _ _ _ _ _ _ _ _ _ _]
        frame "GMU:Remaining:", Default {
          n288 = Match Pattern(string=w793, regular expression="GMU:Remaining:" ("String to match")) -> (match substring=w791:string)  [unwired: 4 out]
          n289 = Empty String/Path?(string/path=w791) -> (empty?=w790:bool)
          n290 = case shown="False" w790 {
            tunnel: [w805 nan] -> w798
            tunnel: w797 -> [w804 _]
            tunnel: w796 -> [w803 _]
            tunnel: w795 -> [w802 _]
            tunnel: w794 -> [w801 _]
            tunnel: w793 -> [w800 _]
            tunnel: [w799 w807] -> w789
            frame False {
              n291 = call "Update_Rem_gas.vi"("Scan Period (s)"=w801, "Gas Remaining in"=w804, "Ch name"=w800, "Ch names"=w802, "Present scan array"=w803) -> ("Gas Remaining out"=w805:dbl, "Comments"=w799:string)  [unwired: 1 out]
            }
            frame True {
              n292 = Current VI's Path() -> (path=w809:path)
              n293 = Path To String(path=w809) -> (string=w808:string)
              n294 = Concatenate Strings(" was not matched in ", w808) -> (w807:string)
            }
          }
        }
        frame "GMU:Source:Meas Q" {
          n295 = call "Calculate_Release_Flowrates.vi"("Ch names"=w820, "Units"=enum16{"Q l/min", "M_dot Kg/min"}."Q l/min", "Present scan array"=w819) -> ("Trace"=w816:dbl, "Carrier"=w817:dbl, "Scan comments"=w818:string)
          n296 = Add(x=w817, y=w816) -> (x+y=w813:dbl)
          n297 = Not Equal To 0?(x=w813) -> (x != 0?=w814:bool)
          n298 = Select(t=w813, s=w814, f=w811) -> (s? t:f=w812:dbl)
        }
        frame "GMU:Detector:Strength" {
          n299 = Unbundle By Name(w822) -> ("C"=w821:dbl)
          n300 = call "Read_value_of_earlier_Ch.vi"("Desired Ch to Read"="GMU:Detector:Meas Current", "Ch names"=w830, "Present scan array"=w831) -> ("Value"=w827:dbl, "Scan comment"=w825:string)  [unwired: 1 in]
          n301 = Greater?(x=w827, y=w821) -> (0:w828:bool)
          n302 = case shown="True" w828 {
            tunnel: w822 -> [_ w843]
            tunnel: w827 -> [_ w838]
            tunnel: [100.0 ("Eng Values") w836] -> w826
            tunnel: ["Fault" w839] -> w823
            frame False {
            }
            frame True {
              n303 = Unbundle By Name(w843) -> ("D"=w834:dbl, "A"=w842:dbl, "B"=w841:dbl)
              n304 = Less?(x=w838, y=w834) -> (x < y?=w837:bool)
              n305 = Build Array(w842, w841) -> (w840:dbl[])
              n306 = call "Polynomial_convert.vi"("Calib constants"=w840, "Voltage"=w838) -> ("Eng Values"=w835:dbl)  [unwired: 4 out]
              n307 = case shown="True" w837 {
                tunnel: ["Saturated" ""] -> w839
                tunnel: [100.0 ("Eng Values") w846] -> w836
                tunnel: w835 -> [_ w846]
                frame False {
                }
                frame True {
                }
              }
            }
          }
          n308 = Concatenate Strings(w825, w823) -> (w824:string)
        }
        frame "GMU:Source:Meas M_dot" {
          n309 = call "Calculate_Release_Flowrates.vi"("Ch names"=w854, "Units"=enum16{"Q l/min", "M_dot Kg/min"}."M_dot Kg/min", "Present scan array"=w853) -> ("Trace"=w850:dbl, "Carrier"=w851:dbl, "Scan comments"=w852:string)
          n310 = Add(x=w851, y=w850) -> (x+y=w848:dbl)
        }
        frame "GMU:Source:Meas Density" {
          n311 = Build Array("GMU:Source:Meas M_dot", "GMU:Source:Meas Q") -> (w860:string[])
          n312 = call "Read_Earlier_Channels.vi"("Present scan array"=w858, "Ch names"=w859, "Desired Channels"=w860) -> ("Scan comments"=w857:string, "Index 0"=w856:dbl, "Index 1"=w855:dbl)  [unwired: 3 out]
          n313 = Not Equal To 0?(x=w856) -> (x != 0?=w864:bool)
          n314 = case shown="False" w864 {
            tunnel: w856 -> [_ w868]
            tunnel: w855 -> [_ w867]
            tunnel: [0.0 w866] -> w863
            frame False {
            }
            frame True {
              n315 = Divide(x=w868, y=w867) -> (x/y=w869:dbl)
              n316 = Multiply(x=w869, y=1000.0) -> (x*y=w866:dbl)
            }
          }
        }
        frame "GMU:Source:Meas Den Ratio" {
          n317 = call "Read_value_of_earlier_Ch.vi"("Desired Ch to Read"="GMU:Source:Meas Density", "Ch names"=w877, "Present scan array"=w878) -> ("Value"=w873:dbl, "Scan comment"=w872:string)  [unwired: 1 in]
          n318 = Equal?(x=w873, y=w871) -> (x = y?=w875:bool)
          n319 = case shown="False" w875 {
            tunnel: w873 -> [w880 _]
            tunnel: [w879 w885] -> w874
            tunnel: w871 -> [_ w885]
            frame False {
              n320 = global read "Gas_management_global.vi" "Release temp (deg C)"() -> (w883:dbl)
              n321 = global read "Gas_management_global.vi" "Atmos Pres (mbars)"() -> (w882:dbl)
              n322 = call "Gas_Density.vi"("Pressure (mbars)"=w882, "Temperature (deg C)"=w883, "Gas Name"="Air") -> ("Density Kg/m3"=w881:dbl)
              n323 = Divide(x=w880, y=w881) -> (x/y=w879:dbl)
            }
            frame True {
            }
          }
        }
        frame "GMU:Source:Meas Strength" {
          n324 = call "Calculate_Release_Flowrates.vi"("Ch names"=w901, "Units"=enum16{"Q l/min", "M_dot Kg/min"}."Q l/min", "Present scan array"=w900) -> ("Trace"=w893:dbl, "Carrier"=w894:dbl, "Scan comments"=w899:string)
          n325 = Equal To 0?(x=w894) -> (x = 0?=w896:bool)
          n326 = Equal To 0?(x=w893) -> (x = 0?=w897:bool)
          n327 = And(x=w896, y=w897) -> (x .and. y?=w895:bool)
          n328 = case shown="False" w895 {
            tunnel: w894 -> [w912 _]
            tunnel: w893 -> [w911 _]
            tunnel: [w910 0.0] -> w889
            frame False {
              n329 = Add(x=w912, y=w911) -> (x+y=w915:dbl)
              n330 = Divide(x=w911, y=w915) -> (x/y=w914:dbl)
              n331 = Multiply(x=w914, y=100.0) -> (x*y=w910:dbl)
            }
            frame True {
            }
          }
          n332 = while {
            tunnel: [w903] -> w886
            tunnel: [w904] -> w888
            tunnel: w889 -> [w909]
            shift-left: _ -> [w903]
            shift-left: _ -> [w908]
            shift-right: [w909] -> _
            stop <- FALSE continue-if-true
            w907 = 6.0 ("y")
            n333 = Less?(x=w908, y=w907) -> (x < y?=w906:bool)
            n334 = Less?(x=w903, y=w907) -> (x < y?=w905:bool)
            n335 = Or(x=w906, y=w905) -> (x .or. y?=w904:bool)
          }
          n336 = Greater?(x=w889, y=7.0) -> (0:w887:bool)
          n337 = And(x=w888, y=w887) -> (x .and. y?=w891:bool)
          n338 = Select(t=w886, s=w891, f=w889) -> (s? t:f=w890:dbl)
        }
        frame "EnFlo Lab:labstrat1:Av Temp" {
          w921 = 0.0 ("Value")
          n339 = for {
            tunnel: w925 -> [w937]
            tunnel: w924 -> [w936]
            shift-right: [w933] -> w922
            shift-left: "" -> [w934]
            shift-right: [w931] -> w920
            shift-left: w921 -> [w930]
            shift-right: [w927] -> w919
            shift-left: w921 -> [w928]
            tunnel: string[] ["EnFlo Lab:labstrat1:Z=4.5m", "EnFlo Lab:labstrat1:Z=3.5m", "EnFlo Lab:labstrat1:Z=2.5m", "EnFlo Lab:labstrat1:Z=1.5m", "EnFlo Lab:labstrat1:Z=0.5m"] -> [w926] mode=indexing
            n340 = call "Read_value_of_earlier_Ch.vi"("Desired Ch to Read"=w926, "Ch names"=w936, "Present scan array"=w937) -> ("Value"=w929:dbl, "Scan comment"=w935:string)  [unwired: 1 in]
            n341 = Concatenate Strings(w934, w935) -> (w933:string)
            n342 = Not A Number/Path/Refnum?(number/path/refnum=w929) -> (NaN/Path/Refnum?=w932:bool)
            n343 = case shown="True" w932 {
              tunnel: [w941 w944] -> w931
              tunnel: w930 -> [w942 w944]
              tunnel: w929 -> [w940 _]
              tunnel: w928 -> [w939 w943]
              tunnel: [w938 w943] -> w927
              frame False {
                n344 = Add(x=w940, y=w942) -> (x+y=w941:dbl)
                n345 = Increment(x=w939) -> (x+1=w938:dbl)
              }
              frame True {
              }
            }
          }
          n346 = Divide(x=w920, y=w919) -> (x/y=w918:dbl)
        }
        frame "EnFlo_Tunnel:Inlet_Temp:St Deviation" {
          n347 = global read "ADAM_Global.vi" "Active Ch names"() -> (w955:string[])
          n348 = Unbundle By Name(w951) -> ("A"=w952:dbl)
          n349 = Less?(x=w952, y=2.0) -> (x < y?=w953:bool)
          n350 = case shown="True" w953 {
            tunnel: w949 -> [_ w991]
            tunnel: w950 -> [_ w990]
            tunnel: string[] ["EnFlo_Tunnel:Inlet_Y=-1500:Z=50", "EnFlo_Tunnel:Inlet_Y=-1000:Z=50", "EnFlo_Tunnel:Inlet_Y=-500:Z=50", "EnFlo_Tunnel:Temp:Inlet_15_Bottom", "EnFlo_Tunnel:Inlet_Y=500:Z=50", "EnFlo_Tunnel:Inlet_Y=1000:Z=50", "EnFlo_Tunnel:Inlet_Y=1500:Z=50", "EnFlo_Tunnel:Inlet_Y=-1500:Z=450", "EnFlo_Tunnel:Inlet_Y=-1000:Z=450", "EnFlo_Tunnel:Inlet_Y=-500:Z=450", "EnFlo_Tunnel:Temp:Inlet_11", "EnFlo_Tunnel:Inlet_Y=500:Z=450", "EnFlo_Tunnel:Inlet_Y=1000:Z=450", "EnFlo_Tunnel:Inlet_Y=1500:Z=450", "EnFlo_Tunnel:Inlet_Y=-1500:Z=950", "EnFlo_Tunnel:Inlet_Y=-1000:Z=950", "EnFlo_Tunnel:Inlet_Y=-500:Z=950", "EnFlo_Tunnel:Temp:Inlet_6", "EnFlo_Tunnel:Inlet_Y=500:Z=950", "EnFlo_Tunnel:Inlet_Y=1000:Z=950", "EnFlo_Tunnel:Inlet_Y=1500:Z=950", "EnFlo_Tunnel:Inlet_Y=-1500:Z=1450", "EnFlo_Tunnel:Inlet_Y=-1000:Z=1450", "EnFlo_Tunnel:Inlet_Y=-500:Z=1450", "EnFlo_Tunnel:Temp:Inlet_1_Top", "EnFlo_Tunnel:Inlet_Y=500:Z=1450", "EnFlo_Tunnel:Inlet_Y=1000:Z=1450", "EnFlo_Tunnel:Inlet_Y=1500:Z=1450", "EnFlo_Tunnel:Setpoint:Inlet_15_Bottom", "EnFlo_Tunnel:Setpoint:Inlet_11", "EnFlo_Tunnel:Setpoint:Inlet_6", "EnFlo_Tunnel:Setpoint:Inlet_1_Top"] ("subarray") -> [w960 w989]
            tunnel: [w958 w987] -> w947
            tunnel: w955 -> [_ w986]
            tunnel: [w961 w983] -> w945
            tunnel: w952 -> [w962 _]
            frame False {
              w968 = FALSE  # All Active Channels
              n351 = Get Date/Time In Seconds() -> (seconds since 1Jan1904=w971:timestamp)
              n352 = To Double Precision Float(number=w971) -> (double precision float=w969:dbl)
              n353 = Subtract(x=w969, y=w962) -> (x-y=w970:dbl)
              n354 = call "Get_ADAM_averages_server.vi"("No of averages"=1, "All Active Channels"=w968, "End time"=w969, "Start time"=w970, "Clients time"=w969, "ADAM Ch Names"=w960) -> ("DBL values"=w966:dbl[][])  [unwired: 4 out]
              n355 = Index Array(array=w966, index (row)=0) -> (element=w963:dbl[])  [unwired: 1 in]
              n356 = Array Subset(array=w963, index=1) -> (w957:dbl[])  [unwired: 1 in]
              n357 = call "Normalise Inlet Temps array.vi"("Temps plus setpoints"=w957) -> ("Normalised Temps"=w956:dbl[])
              n358 = for {
                tunnel: w956 -> [w977] mode=indexing
                tunnel: [w977] -> w961 mode=indexing if=w975
                tunnel: w960 -> [w974] mode=indexing
                shift-right: [w972] -> w958
                shift-left: "" -> [w973]
                n359 = Not A Number/Path/Refnum?(number/path/refnum=w977) -> (NaN/Path/Refnum?=w976:bool)
                n360 = Not(x=w976) -> (.not. x?=w975:bool)
                n361 = case shown="False" w975 {
                  tunnel: w974 -> [w980 _]
                  tunnel: w973 -> [w979 w982]
                  tunnel: [w978 w982] -> w972
                  frame False {
                    n362 = Format Into String(format string="Channel \"%s\" is not currently active.\n", initial string=w979, w980) -> (resulting string=w978:string)  [unwired: 1 in, 1 out]
                  }
                  frame True {
                  }
                }
              }
            }
            frame True {
              n363 = for {
                tunnel: w991 -> [w1005]
                tunnel: w990 -> [w1004]
                tunnel: w989 -> [w1001] mode=indexing
                shift-right: [w1002] -> w987
                shift-left: "" -> [w1003]
                tunnel: w986 -> [w996]
                tunnel: [w995] -> w985 mode=indexing
                n364 = call "Read_value_of_earlier_Ch.vi"("Desired Ch to Read"=w1001, "Ch names"=w1005, "Present scan array"=w1004) -> ("Value"=w999:dbl, "Scan comment"=w998:string)  [unwired: 1 in]
                n365 = Not A Number/Path/Refnum?(number/path/refnum=w999) -> (NaN/Path/Refnum?=w1000:bool)
                n366 = case shown="False" w1000 {
                  tunnel: w1001 -> [w1008 _]
                  tunnel: [w1011 w1021] -> w995
                  tunnel: w999 -> [w1010 w1021]
                  tunnel: [w1013 w1020] -> w997
                  tunnel: w998 -> [w1012 w1020]
                  tunnel: w996 -> [w1009 _]
                  frame False {
                    n367 = Search 1D Array(1D array=w1009, element=w1008) -> (index of element=w1006:i32)  [unwired: 1 in]
                    n368 = Greater Or Equal To 0?(x=w1006) -> (x >= 0?=w1007:bool)
                    n369 = case shown="False" w1007 {
                      tunnel: w1008 -> [w1017 _]
                      tunnel: [w1016 w1019] -> w1013
                      tunnel: w1012 -> [_ w1019]
                      tunnel: [nan w1018] -> w1011
                      tunnel: w1010 -> [_ w1018]
                      frame False {
                        n370 = Format Into String(format string="Channel \"%s\" is not currently active.\n", w1017) -> (resulting string=w1016:string)  [unwired: 2 in, 1 out]
                      }
                      frame True {
                      }
                    }
                  }
                  frame True {
                  }
                }
                n371 = Concatenate Strings(w1003, w997) -> (w1002:string)
              }
              n372 = call "Normalise Inlet Temps array.vi"("Temps plus setpoints"=w985) -> ("Normalised Temps"=w984:dbl[])
              n373 = for {
                tunnel: w984 -> [w993] mode=indexing
                tunnel: [w993] -> w983 mode=indexing if=w992
                n374 = Not A Number/Path/Refnum?(number/path/refnum=w993) -> (NaN/Path/Refnum?=w994:bool)
                n375 = Not(x=w994) -> (.not. x?=w992:bool)
              }
            }
          }
          n376 = call <vilib>:"Std Deviation and Variance.vi"("X"=w945) -> ("standard deviation"=w946:dbl)  [unwired: 1 in, 2 out]
        }
        frame "EnFlo Lab:labstrat1:Delta T" {
          n377 = Build Array("EnFlo Lab:labstrat1:Z=4.5m", "EnFlo Lab:labstrat1:Z=0.5m") -> (w1029:string[])
          n378 = call "Read_Earlier_Channels.vi"("Present scan array"=w1025, "Ch names"=w1026, "Desired Channels"=w1029) -> ("Scan comments"=w1024:string, "Index 0"=w1023:dbl, "Index 1"=w1022:dbl)  [unwired: 3 out]
          n379 = Subtract(x=w1023, y=w1022) -> (x-y=w1030:dbl)
        }
        frame "EnFlo_Tunnel:Inlet:K_Factor" {
          n380 = call "Read_value_of_earlier_Ch.vi"("Desired Ch to Read"="EnFlo_Tunnel:Speed:Dem Velocity", "Ch names"=w1036, "Present scan array"=w1037) -> ("Value"=w1032:dbl)  [unwired: 1 in, 1 out]
          n381 = Build Array("EnFlo_Tunnel:Pressure:Static", "EnFlo_Tunnel:Reference:Velocity", "Froude:NPL:Atmos_Press", "EnFlo_Tunnel:Inlet_Temp:Average") -> (w1049:string[])
          n382 = call "Read_Earlier_Channels.vi"("Present scan array"=w1037, "Ch names"=w1036, "Desired Channels"=w1049) -> ("Scan comments"=w1046:string, "Index 0"=w1041:dbl, "Index 1"=w1039:dbl, "Index 2"=w1042:dbl, "Index 3"=w1043:dbl)  [unwired: 1 out]
          n383 = Greater?(x=w1039, y=0.8) -> (0:w1034:bool)
          n384 = while {
            shift-right: [w1053] -> _
            shift-left: _ -> [_]
            shift-left: _ -> [_]
            shift-left: _ -> [_]
            shift-left: _ -> [_]
            shift-left: _ -> [_]
            shift-left: _ -> [_]
            shift-left: _ -> [_]
            shift-left: _ -> [_]
            shift-left: _ -> [_]
            shift-left: _ -> [_]
            shift-left: _ -> [w1052]
            tunnel: w1032 -> [w1053]
            tunnel: [w1051] -> w1031
            stop <- TRUE stop-if-true
            n385 = Equal?(x=w1053, y=w1052) -> (x = y?=w1051:bool)
          }
          n386 = And(x=w1031, y=w1034) -> (x .and. y?=w1033:bool)
          n387 = case shown="True" w1033 {
            tunnel: w1043 -> [_ w1059]
            tunnel: w1042 -> [_ w1058]
            tunnel: w1039 -> [_ w1057]
            tunnel: w1041 -> [_ w1056]
            tunnel: [nan w1055] -> w1040
            frame False {
            }
            frame True {
              n388 = formula code="Rho=(Patmos*100)/(287*(T+273));\nDyn_Pres=0.5*Rho*U*U;\nK=(-Pstatic/Dyn_Pres)-1;"("Pstatic"=w1056, "Patmos"=w1058, "T"=w1059, "U"=w1057) -> ("K"=w1055:dbl)  [unwired: 2 out]
            }
          }
        }
        frame "EnFlo_Tunnel:Chilled Water:Valve Dem Pos" {
          n389 = Get Date/Time In Seconds() -> (seconds since 1Jan1904=w1061:timestamp)
          n390 = Concatenate Strings(w1062, " last updated") -> (w1070:string)
          n391 = To Double Precision Float(number=w1061) -> (double precision float=w1060:dbl)
          n392 = Unbundle By Name(w1068) -> ("A"=w1067:dbl)
          n393 = call "Remember_value.vi"("Mode"=Remember_value_mode."Read only", "Ch name"=w1070) -> ("Output Value"=w1069:dbl)  [unwired: 1 in]
          n394 = Subtract(x=w1060, y=w1069) -> (x-y=w1066:dbl)
          n395 = Greater?(x=w1066, y=w1067) -> (0:w1065:bool)
          n396 = Not A Number/Path/Refnum?(number/path/refnum=w1066) -> (NaN/Path/Refnum?=w1064:bool)
          n397 = Or(x=w1064, y=w1065) -> (x .or. y?=w1063:bool)
          n398 = case shown="True" w1063 {
            tunnel: w1077 -> [w1078 w1080]
            tunnel: [w1078 w1097] -> w1076
            tunnel: w1075 -> [_ w1089]
            tunnel: w1074 -> [_ w1090]
            tunnel: ["" w1095] -> w1073
            tunnel: w1070 -> [_ w1085]
            tunnel: w1060 -> [_ w1081]
            frame False {
            }
            frame True {
              n399 = call "Read_value_of_earlier_Ch.vi"("Desired Ch to Read"="EnFlo_Tunnel:Chiller_Pump:Enable", "Ch names"=w1090, "Present scan array"=w1089) -> ("Value"=w1088:dbl)  [unwired: 1 in, 1 out]
              n400 = Build Array("EnFlo_Tunnel:Chilled Water:Dem Temp", "EnFlo_Tunnel:Chilled Water:Supply", "EnFlo_Tunnel:Chiller_Pump:Running") -> (w1096:string[])
              n401 = call "Read_Earlier_Channels.vi"("Present scan array"=w1089, "Ch names"=w1090, "Desired Channels"=w1096) -> ("Scan comments"=w1095:string, "Index 0"=w1094:dbl, "Index 1"=w1093:dbl, "Index 2"=w1083:dbl)  [unwired: 2 out]
              n402 = Greater?(x=w1088, y=0.5) -> (0:w1086:bool)
              n403 = Greater?(x=w1083, y=0.5) -> (0:w1082:bool)
              n404 = case shown="True" w1082 {
                tunnel: [w1112 w1120] -> w1097
                tunnel: w1094 -> [_ w1122]
                tunnel: w1093 -> [_ w1121]
                tunnel: w1081 -> [_ w1119]
                tunnel: w1086 -> [w1103 _]
                tunnel: w1085 -> [_ w1118]
                tunnel: w1080 -> [_ w1116]
                frame False {
                  n405 = Seconds To Date/Time() -> (date time rec=w1100:T16)  [unwired: 2 out]
                  n406 = Unbundle By Name(w1100) -> ("day of week"=w1107:i32, "hour"=w1109:i32)
                  n407 = Less?(x=w1109, y=3) -> (x < y?=w1104:bool)
                  n408 = Equal?(x=7, y=w1107) -> (x = y?=w1105:bool)
                  n409 = And(x=w1105, y=w1104) -> (x .and. y?=w1102:bool)
                  n410 = case shown="True" w1103 {
                    tunnel: w1102 -> [w1113 w1115]
                    tunnel: [w1113 w1114] -> w1101
                    frame False {
                    }
                    frame True {
                      n411 = Not(x=w1115) -> (.not. x?=w1114:bool)
                    }
                  }
                  n412 = Select(t=0.0, s=w1101, f=100.0) -> (s? t:f=w1112:dbl)
                }
                frame True {
                  w1124 = 100.0  # Max
                  w1125 = 0.0  # Min
                  n413 = call "PID.vi"("Present Value"=w1121, "Previous Scan Value"=w1116, "Setpoint"=w1122) -> ("Dem Output"=w1123:dbl)
                  n414 = In Range and Coerce(upper limit=w1124, x=w1123, lower limit=w1125) -> (coerced(x)=w1120:dbl)  [unwired: 1 out]
                  n415 = call "Remember_value.vi"("Mode"=Remember_value_mode."Read and Write", "Input Value"=w1119, "Ch name"=w1118) -> ()  [unwired: 1 out]
                }
              }
            }
          }
        }
        frame "EnFlo_Tunnel:Hydrosonic:Integral" {
          n416 = Build Array("EnFlo_Tunnel:Reference:Velocity", "Hydrosonic:Transducer:Setting") -> (w1135:string[])
          n417 = call "Read_Earlier_Channels.vi"("Present scan array"=w1136, "Ch names"=w1134, "Desired Channels"=w1135) -> ("Scan comments"=w1128:string, "Index 0"=w1133:dbl, "Index 1"=w1127:dbl)  [unwired: 3 out]
          n418 = Greater?(x=w1133, y=0.5) -> (0:w1131:bool)
          n419 = case shown="True" w1131 {
            tunnel: w1130 -> [w1139 w1147]
            tunnel: [w1139 w1146] -> w1129
            tunnel: w1127 -> [_ w1145]
            tunnel: w1126 -> [_ w1144]
            frame False {
            }
            frame True {
              w1142 = 8640000.0  # Seconds per day x 100
              n420 = Multiply(x=w1145, y=w1144) -> (x*y=w1143:dbl)
              n421 = Divide(x=w1143, y=w1142) -> (x/y=w1141:dbl)
              n422 = Not A Number/Path/Refnum?(number/path/refnum=w1141) -> (NaN/Path/Refnum?=w1140:bool)
              n423 = case shown="False" w1140 {
                tunnel: w1147 -> [w1150 w1151]
                tunnel: [w1149 w1151] -> w1146
                tunnel: w1141 -> [w1148 _]
                frame False {
                  n424 = Add(x=w1148, y=w1150) -> (x+y=w1149:dbl)
                }
                frame True {
                }
              }
            }
          }
        }
        frame "EnFlo_Tunnel:Days Run at:2.5m/s" {
          n425 = Build Array("EnFlo_Tunnel:Reference:Velocity") -> (w1160:string[])
          n426 = call "Read_Earlier_Channels.vi"("Present scan array"=w1161, "Ch names"=w1159, "Desired Channels"=w1160) -> ("Scan comments"=w1154:string, "Index 0"=w1152:dbl)  [unwired: 4 out]
          n427 = Greater?(x=w1152, y=0.5) -> (0:w1157:bool)
          n428 = case shown="True" w1157 {
            tunnel: w1156 -> [w1163 w1171]
            tunnel: [w1163 w1170] -> w1155
            tunnel: w1152 -> [_ w1169]
            tunnel: w1153 -> [_ w1168]
            frame False {
            }
            frame True {
              w1166 = 216000.0  # Seconds per day x 2.5
              n429 = Multiply(x=w1169, y=w1168) -> (x*y=w1167:dbl)
              n430 = Divide(x=w1167, y=w1166) -> (x/y=w1165:dbl)
              n431 = Not A Number/Path/Refnum?(number/path/refnum=w1165) -> (NaN/Path/Refnum?=w1164:bool)
              n432 = case shown="True" w1164 {
                tunnel: w1171 -> [w1174 w1175]
                tunnel: [w1173 w1175] -> w1170
                tunnel: w1165 -> [w1172 _]
                frame False {
                  n433 = Add(x=w1172, y=w1174) -> (x+y=w1173:dbl)
                }
                frame True {
                }
              }
            }
          }
        }
        frame "Complete:Scan:Period" {
          n434 = while {
            tunnel: [w1185] -> w1178
            tunnel: [w1192] -> w1180
            shift-left: _ -> [w1192]
            shift-right: [w1193] -> w1181
            tunnel: w1177 -> [w1189]
            tunnel: [w1184] -> w1176
            stop <- FALSE continue-if-true
            w1184 = 10.0 ("Averaging time (mins)")
            n435 = Build Array(w1189) -> (w1188:string[])
            n436 = call "Get_Channel_averages.vi"("Desired Ch Names"=w1188, "Averaging time (mins)"=w1184) -> ("number"=w1187:dbl[])  [unwired: 1 in, 2 out]
            n437 = Index Array(array=w1187, index=0) -> (element=w1185:dbl)
            n438 = Greater?(x=w1185, y=20.0) -> (0:w1193:bool)
          }
          n439 = Compound Arithmetic op=AND(w1181, invert w1180) -> (w1179:bool)
          n440 = case shown="True" w1179 {
            tunnel: w1178 -> [_ w1199]
            tunnel: w1176 -> [_ w1194]
            frame False {
            }
            frame True {
              n441 = Format Into String(format string="Warning! The average scan period on the ADAM Scan table is %.1f seconds over the last %d minutes." ("Format String"), w1199, w1194) -> (resulting string=w1197:string)  [unwired: 2 in, 1 out]
              n442 = call "Server_Emails.vi"("Message"=w1197, "Contact All clients?"=TRUE, "Subject"="Scan Period") -> ()  [unwired: 2 in, 3 out]
            }
          }
        }
        frame "GMU:Source:Est Time" {
          # "NaN's"
          # "Est?"
          # "Inband?"
          n443 = stacked-sequence {
            seq-local: [w1206 _ _ _] -> [_ _ w1253 _]
            seq-local: [_ w1218 _ _] -> [_ _ w1250 _]
            seq-local: [_ w1219 _ _] -> [_ _ w1248 _]
            seq-local: [_ _ w1255 _] -> [_ _ _ w1271]
            seq-local: [w1210 _ _ _] -> [_ _ w1252 _]
            seq-local: [_ w1217 _ _] -> [_ _ _ w1267]
            tunnel: w1205 -> [w1212 w1220 w1258 _]
            tunnel: w1204 -> [w1211 w1221 w1259 _]
            tunnel: [_ _ w1251 _] -> w1203
            tunnel: [_ _ _ w1270] -> w1202
            tunnel: w1201 -> [_ _ _ w1269]
            tunnel: w1200 -> [_ _ _ w1268]
            frame #0 {
              n444 = Build Array("GMU:Source:Density Ratio", "GMU:Source:Dem Strength", "GMU:Source:Dem Q") -> (w1213:string[])
              n445 = call "Read_Earlier_Channels.vi"("Present scan array"=w1211, "Ch names"=w1212, "Desired Channels"=w1213) -> ("Scan comments"=w1210:string, "Index 0"=w1209:dbl, "Index 1"=w1208:dbl, "Index 2"=w1207:dbl)  [unwired: 2 out]
              n446 = Build Array(w1209, w1208, w1207) -> (w1206:dbl[])
            }
            frame #1 {
              n447 = for {
                N: 2 -> [_]
                tunnel: w1221 -> [w1231]
                tunnel: w1220 -> [w1232]
                tunnel: [w1230] -> w1218 mode=indexing
                tunnel: [w1237] -> w1219 mode=indexing
                tunnel: [w1236] -> w1217 mode=indexing
                i -> [w1242]
                w1241 = 23.0  # %
                n448 = case shown="1" w1242 {
                  tunnel: ["GMU:Source:Meas Q" "GMU:Source:Meas Strength"] -> w1235
                  tunnel: ["GMU:Source:Dem Q" "GMU:Source:Dem Strength"] -> w1234
                  frame 0, Default {
                  }
                  frame 1 {
                  }
                }
                n449 = Build Array(w1234, w1235) -> (w1233:string[])
                n450 = call "Read_Earlier_Channels.vi"("Present scan array"=w1231, "Ch names"=w1232, "Desired Channels"=w1233) -> ("Scan comments"=w1230:string, "Index 0"=w1228:dbl, "Index 1"=w1229:dbl)  [unwired: 3 out]
                n451 = Not A Number/Path/Refnum?(number/path/refnum=w1229) -> (NaN/Path/Refnum?=w1236:bool)
                n452 = Subtract(x=w1229, y=w1228) -> (x-y=w1227:dbl)
                n453 = Greater Than 0?(x=w1228) -> (x > 0?=w1238:bool)
                n454 = Less?(x=w1227, y=0.05) -> (x < y?=w1224:bool)
                n455 = call "In_Range_check.vi"("%"=w1241, "Mode"=In_Range."%", "Value"=w1229, "Setpoint"=w1228) -> ("In Range"=w1225:bool)  [unwired: 1 in, 2 out]
                n456 = Or(x=w1225, y=w1224) -> (x .or. y?=w1223:bool)
                n457 = And(x=w1223, y=w1238) -> (x .and. y?=w1239:bool)
                n458 = Compound Arithmetic op=OR(w1239, invert w1238, w1236) -> (w1237:bool)
              }
            }
            frame #2 {
              n459 = while {
                tunnel: [w1266] -> w1254
                tunnel: w1253 -> [w1265]
                shift-left: _ -> [w1266]
                shift-right: [w1265] -> _
                stop <- FALSE continue-if-true
              }
              n460 = Equal?(x=w1253, y=w1254) -> (x = y?=w1260:bool)
              n461 = call "Read_value_of_earlier_Ch.vi"("Desired Ch to Read"="GMU:Source:Dem Q", "Ch names"=w1258, "Present scan array"=w1259) -> ("Value"=w1256:dbl)  [unwired: 1 in, 1 out]
              n462 = Greater Than 0?(x=w1256) -> (x > 0?=w1263:bool)
              n463 = And Array Elements(Boolean array=w1248) -> (logical AND=w1247:bool)
              n464 = Select(t=w1247, s=w1263, f=TRUE) -> (s? t:f=w1261:bool)
              n465 = Compound Arithmetic op=AND(w1260, w1261) -> (w1255:bool)
              n466 = Concatenate Strings(w1250) -> (w1249:string)
              n467 = Concatenate Strings(w1249, w1252) -> (w1251:string)
            }
            frame #3 {
              n468 = case shown="True" w1271 {
                tunnel: [0.0 w1273] -> w1270
                tunnel: w1269 -> [_ w1278]
                tunnel: w1268 -> [_ w1274]
                tunnel: w1267 -> [_ w1277]
                frame False {
                }
                frame True {
                  n469 = Or Array Elements(Boolean array=w1277) -> (logical OR=w1276:bool)
                  n470 = Add(x=w1278, y=w1274) -> (x+y=w1275:dbl)
                  n471 = Select(t=w1274, s=w1276, f=w1275) -> (s? t:f=w1273:dbl)
                }
              }
            }
          }
        }
      }
    }
    frame "Vaisala" {
      n472 = Unbundle By Name(w1285) -> ("Main"=w1281:i32, "Ch."=w1282:i32, "Port Name"=w1283:string)
      n473 = call "HMP231.vi"("Channel Name"=w1284, "Port Name"=w1283, "Channel"=w1282, "Address"=w1281) -> ("Output"=w1279:dbl, "Status note"=w1280:string)  [unwired: 2 out]
    }
    frame "WEST" {
    }
    frame "Web Client" {
      w1297 = 7200.0  # 2 Hours in Seconds
      n474 = Concatenate Strings(w1306, ":Last read" ("Substring")) -> (w1304:string)
      n475 = call "Remember_value.vi"("Mode"=Remember_value_mode."Read only", "Ch name"=w1304) -> ("Output Value"=w1303:dbl)  [unwired: 1 in]
      n476 = Not A Number/Path/Refnum?(number/path/refnum=w1303) -> (NaN/Path/Refnum?=w1301:bool)
      n477 = Get Date/Time In Seconds() -> (seconds since 1Jan1904=w1296:timestamp)
      n478 = To Double Precision Float(number=w1296) -> (double precision float=w1294:dbl)
      n479 = Subtract(x=w1294, y=w1303) -> (x-y=w1309:dbl)
      n480 = Greater?(x=w1309, y=1800.0) -> (0:w1302:bool)
      n481 = Or(x=w1302, y=w1301) -> (x .or. y?=w1288:bool)
      n482 = case shown="True" w1288 {
        frame False {
        }
        frame True {
          n483 = global read "Constants_global.vi" "EnFlo SW Folder"() -> (w1312:path)
          n484 = Build Path(base path=w1312, name or relative path=path "ADAM Server/Sub VI's/Web_Client.vi") -> (appended path=w1311:path)
          n485 = Open VI Reference(vi path=w1311) -> (vi reference=w1316:refnum<vi>, error out=w1317:errorcluster)  [unwired: 1 in, 4 out]
          n486 = property class="VI"(reference=w1316, error in=w1317) -> (reference out=w1319:refnum<vi>, error out=w1320:errorcluster, "Front Panel Window:Open"=w1318:bool)
          n487 = case shown="False" w1318 {
            tunnel: w1319 -> [w1326 w1329]
            tunnel: w1320 -> [w1325 w1328]
            tunnel: [w1324 w1329] -> w1321
            tunnel: [w1323 w1328] -> w1322
            frame False {
              n488 = property class="VI"(reference=w1326, error in=w1325, "Front Panel Window:Open"=TRUE) -> (reference out=w1324:refnum<vi>, error out=w1323:errorcluster)
            }
            frame True {
            }
          }
          n489 = invoke class="VI" method="Run VI"(reference=w1321, error in=w1322, "Wait until done"=FALSE, "Auto Dispose Ref"=TRUE) -> ()  [unwired: 1 in, 5 out]
        }
      }
      n490 = Concatenate Strings(w1306, ":value time" ("Substring")) -> (w1290:string)
      n491 = call "Remember_value.vi"("Mode"=Remember_value_mode."Read only", "Ch name"=w1306) -> ("Output Value"=w1310:dbl)  [unwired: 1 in]
      n492 = call "Remember_value.vi"("Mode"=Remember_value_mode."Read only", "Ch name"=w1290) -> ("Output Value"=w1295:dbl)  [unwired: 1 in]
      n493 = Subtract(x=w1294, y=w1295) -> (x-y=w1293:dbl)
      n494 = Greater?(x=w1293, y=w1297) -> (0:w1300:bool)
      n495 = case shown="True" w1300 {
        tunnel: w1293 -> [_ w1335]
        tunnel: 3600.0 ("y") -> [_ w1334]
        tunnel: ["" w1332] -> w1299
        frame False {
        }
        frame True {
          n496 = Divide(x=w1335, y=w1334) -> (x/y=w1331:dbl)
          n497 = Format Into String(format string="Value is %d hours old." ("Format String"), w1331) -> (resulting string=w1332:string)  [unwired: 2 in, 1 out]
        }
      }
    }
    frame "X10" {
      (unwired) 1 items=["-----", "A", "B", "C", "D", "E", "F", "G", "H", "I", "J", "K", "L", "M", "N", "O", "P"] ("House Code")
      n498 = Greater Than 0?(x=w1340) -> (x > 0?=w1339:bool)
      n499 = Unbundle By Name(w1345) -> ("Port Name"=w1342:string, "Main"=w1343:i32, "Ch."=w1344:i32)
      n500 = call "X10control.vi"("Port Name"=w1342, "Power Request (ON)"=w1339, "House Code"=w1343, "Unit No."=w1344) -> ()  [unwired: 6 out]
      n501 = Select(t=1.0, s=w1339, f=0.0) -> (s? t:f=w1336:dbl)
    }
  }
  "Output" <- w8
  "Scan comment" <- w5
